vi "数据采集传输系统.vi"() -> ()   [LabVIEW 2016, in "数据传输系统.lvlib"]
uses:
  <vilib>/Utility/miscctls.llb/LVPointTypeDef.ctl
  <vilib>/Utility/config.llb/Read Key (String).vi
  <vilib>/Utility/config.llb/Read Key (Boolean).vi
  <vilib>/Utility/config.llb/Read Key (I32).vi
  <vilib>/Utility/config.llb/Write Key (String).vi
  <vilib>/Utility/config.llb/Write Key (U32).vi
  <vilib>/Utility/config.llb/Write Key (Boolean).vi
  <vilib>/Utility/config.llb/Write Key (I32).vi
  <vilib>/Utility/config.llb/NI_LVConfig.lvlib
  data/FreeMem.dll
  <vilib>/ptbypt/NI_PtbyPt.lvlib
panel:
  in  "实时数据发送时间间隔/min":i32=1
  in  "数据组合发送":bool
  in  "日志、参数发送":bool
  in  "2011发送":bool
  in  "判断数据反馈":bool
  in  "数据发送协议":enum16{"2005-212协议", "2017-212协议"}(ring)=enum."2017-212协议"
  in  "数据发送通道":enum16{"TCP", "VISA"}(ring)
  in  "baud rate":u32=9600 caption="波特率"
  in  "VISA resource name":refnum<visa-resource-name> caption="VISA资源名称"
  in  "查询质控数据起始时间":bool
  in  "返回主界面":bool
  out "零点核查索引起始时间":string
  out "跨度核查索引起始时间":string
  out "加标回收索引起始时间":string
  out "标样核查索引起始时间":string
  out "数据接收超时指示灯":bool
  in  "重发时间":T1(ring)
  in  "重发日期":T2(ring)
  in  "锁":bool
  in  "开机启动":bool
  in  "确定更改起始时间":bool
  in  "更改起始时间":bool
  in  "数据发送起始时间":timestamp format="%<%.3X\n%Y/%m/%d>T"
  in  "每周自动重发":bool=TRUE
  in  "确定":bool
  in  "返回":bool
  in  "PW":string
  in  "MN":string
  in  "PORT":string
  in  "IP":string
  in  "站点设备":string
  in  "站点名称":string
  out "设置超时时间/min":i32=1
  out "空闲时间/s":string
  out "状态信息":T3={"1st Error to Convert "=63, "步骤 "=enum."打开连接", "元素"="实时数据", "TCP服务端掉线计数"=4, "TCP掉线时间节点"="2019/05/08 15:24:17"} {"1st Error to Convert" items=["无错误", "参数错误", "内存已满", "超出区域", "文件结束", "文件已打开", "一般文件IO错误", "未找到文件", "文件权限错误", "磁盘已满", "路径副本", "打开过多文件", "未启用", "未找到资源文件", "无法添加资源", "未找到资源", "未找到图像", "图像内存错误", "画笔不存在", "配置错误类型", "配置未找到解析段", "配置解析错误", "配置内存错误", "错误外部代码格式", "错误外部代码偏移量", "外部代码不存在", "空窗口", "销毁窗口错误", "空菜单", "打印已中止", "错误打印记录", "打印驱动程序错误", "打印时窗口错误", "打印时内存错误", "打印对话框错误", "一般打印错误", "无效设备引用句柄", "设备未找到", "设备参数错误", "设备单位错误", "无法打开设备", "设备调用已中止", "一般错误", "用户已取消", "对象ID过低", "对象ID过高", "对象不在堆中", "未知的堆", "错误DefProc ID", "DefProc不在表格中", "范围外信息", "空方法", "未知信息", "不支持管理器调用", "错误地址", "连接过程中", "连接超时", "连接过程中", "不支持网络属性", "网络错误", "正在使用的地址", "系统缺少内存", "连接已中止", "连接已拒绝", "连接未建立", "连接已建立", "连接已关闭", "初始化错误（交互应用程序管理器）", "错误事件发生", "等待无约束事件发生处理程序", "事件发生队列溢出", "错误路径", "未发出信号量", "未识别类型（交互应用程序管理器）"]}
  out "系统时间":string
  out "实时小时数据上传":bool
  out "系统状态改变":bool
  out "软件版本":string
  out "掉线指示":bool
  out "核查数据上传":bool
  out "通信状态":bool
  out "配置信息":T4
  in  "参数配置":bool
  out "查询数据发送":bool
  out "读取报文显示":string
  out "发送报文显示":string
  out "心跳包":bool
  in  "参数数值":T5={"CODMn"=TRUE, "CODCr"=TRUE, "DO"=TRUE, "铜"=TRUE, "PH"=TRUE, "氨氮"=TRUE, "比电导率"=TRUE, "水温"=TRUE, "盐度(海水)"=TRUE, "浊度"=TRUE, "总氮"=TRUE, "总磷"=TRUE, "叶绿素a"=TRUE, "藻密度"=TRUE, "水位"=TRUE, "流速"=TRUE, "瞬时流量"=TRUE, "累积流量"=TRUE}
  in  "系统编码选择框":string(combo)="地表水质量监测"
  out "主队列输出":refnum<queue>
  in  "TCP掉线时间节点":string
  out "TCP服务端掉线计数":i32
  out "元素":string
  out "步骤":T6(ring)
  out "1st Error to Convert":i32(ring)=56 items=["无错误", "参数错误", "内存已满", "超出区域", "文件结束", "文件已打开", "一般文件IO错误", "未找到文件", "文件权限错误", "磁盘已满", "路径副本", "打开过多文件", "未启用", "未找到资源文件", "无法添加资源", "未找到资源", "未找到图像", "图像内存错误", "画笔不存在", "配置错误类型", "配置未找到解析段", "配置解析错误", "配置内存错误", "错误外部代码格式", "错误外部代码偏移量", "外部代码不存在", "空窗口", "销毁窗口错误", "空菜单", "打印已中止", "错误打印记录", "打印驱动程序错误", "打印时窗口错误", "打印时内存错误", "打印对话框错误", "一般打印错误", "无效设备引用句柄", "设备未找到", "设备参数错误", "设备单位错误", "无法打开设备", "设备调用已中止", "一般错误", "用户已取消", "对象ID过低", "对象ID过高", "对象不在堆中", "未知的堆", "错误DefProc ID", "DefProc不在表格中", "范围外信息", "空方法", "未知信息", "不支持管理器调用", "错误地址", "连接过程中", "连接超时", "连接过程中", "不支持网络属性", "网络错误", "正在使用的地址", "系统缺少内存", "连接已中止", "连接已拒绝", "连接未建立", "连接已建立", "连接已关闭", "初始化错误（交互应用程序管理器）", "错误事件发生", "等待无约束事件发生处理程序", "事件发生队列溢出", "错误路径", "未发出信号量", "未识别类型（交互应用程序管理器）"]
  out "QN":string
  out "时间QN":string
  out "系统编码ST":string
  out "命令编码CN":string
  out "密码PW":string
  out "设备编码MN":string
  out "拆分包及应答Flag":string
  out "数据":string
  in  "实时数据参数选择框":T7={"水样测量数据"=FALSE, "零点核查数据"=TRUE, "跨度核查数据"=TRUE, "加标回收数据"=TRUE, "平行样数据"=FALSE, "标样核查"=TRUE, "集成干预测试"=TRUE}
  out "数据输出":string
  in  "table元素":string
  out "空闲时间":dbl
  # "数 据 采 集 传 输 系 统"
  # "读取的参数区"
  # "水样测量数据"
  # "空白测试数据"
  # "跨度核查数据"
  # "加标回收数据"
  # "平行样数据"
  # "标样核查"
  # "集成干预测试"
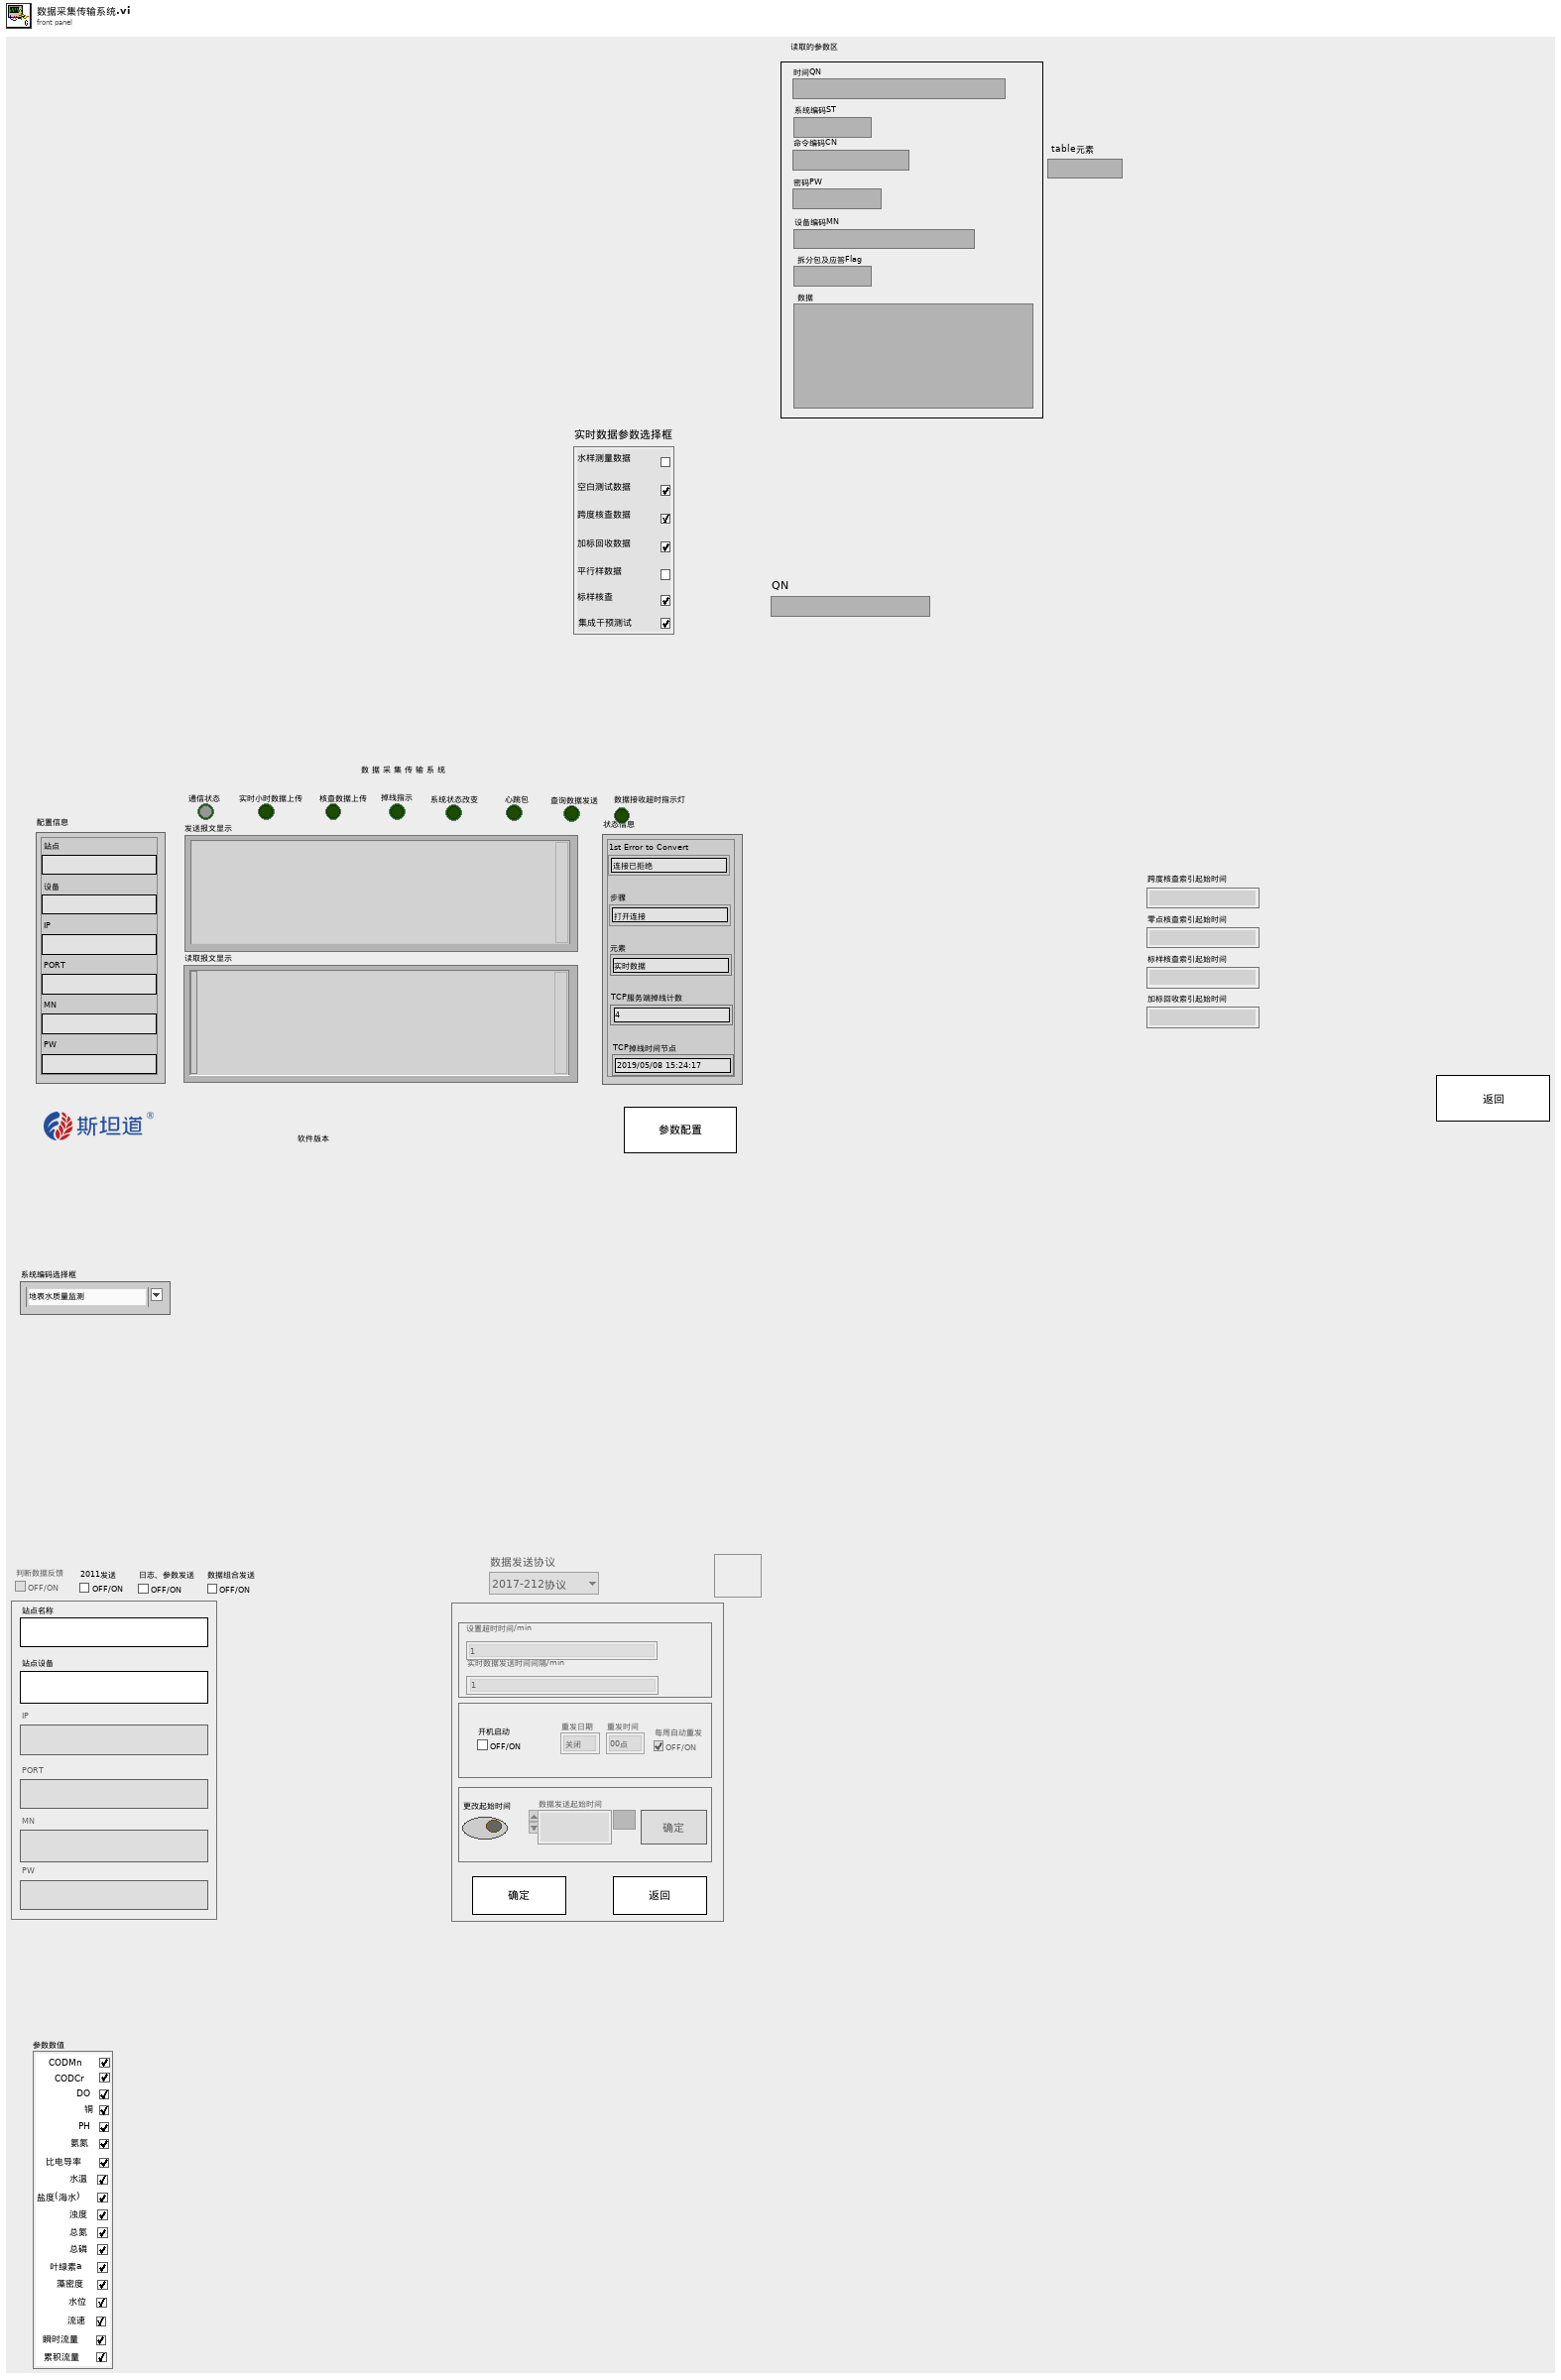
[diagram p1: front panel]
types:
  T1 = enum16{"00点", "01点", "02点", "03点", "04点", "05点", "06点", "07点", "08点", "09点", "10点", "11点", "12点", "13点", "14点", "15点", "16点", "17点", "18点", "19点", "20点", "21点", "22点", "23点"}
  T2 = enum16{"关闭", "星期日", "星期一", "星期二", "星期三", "星期四", "星期五", "星期六"}
  T3 = cluster{"1st Error to Convert ":i32, "步骤 ":enum16{"初始化", "打开连接", "表格比对", "发送数据", "读取数据", "数据处理"}, "元素":string, "TCP服务端掉线计数":i32, "TCP掉线时间节点":string}
  T4 = cluster{"站点":string, "设备":string, "IP":string, "PORT":string, "MN":string, "PW":string}
  T5 = cluster{"CODMn":bool, "CODCr":bool, "DO":bool, "铜":bool, "PH":bool, "氨氮":bool, "比电导率":bool, "水温":bool, "盐度(海水)":bool, "浊度":bool, "总氮":bool, "总磷":bool, "叶绿素a":bool, "藻密度":bool, "水位":bool, "流速":bool, "瞬时流量":bool, "累积流量":bool}
  T6 = enum16{"初始化", "打开连接", "表格比对", "发送数据", "读取数据", "数据处理"}
  T7 = cluster{"水样测量数据":bool, "零点核查数据":bool, "跨度核查数据":bool, "加标回收数据":bool, "平行样数据":bool, "标样核查":bool, "集成干预测试":bool}
  T8 = typedef "NI_LVConfig.lvlib/Config Data RefNum.ctl" = refnum<k1>
  T9 = typedef "LVDateTimeRec.ctl" = cluster{"秒数的小数部分":dbl, "秒":i32, "分":i32, "时":i32, "日":i32, "月":i32, "年":i32, "天数（周）":i32, "天数（年）":i32, "DST":i32}
  T10 = enum8{"Enabled", "Disabled", "Disabled and Grayed Out"}
  T11 = typedef "LVPointTypeDef.ctl" = cluster{"Horizontal":i16, "Vertical":i16}
  T12 = enum16{"水样测试", "小时数据", "日志信息", "报警信息", "零点核查", "标样核查", "平行样", "加标回收"}
  T13 = typedef "imagedata.ctl" = cluster{"image type":i32, "image depth":i32, "image":u8[], "mask":u8[], "colors":u32[], "Rectangle":cluster{"left":i16, "top":i16, "right":i16, "bottom":i16}}
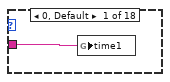
[diagram p5: hidden frame]
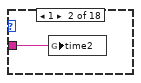
[diagram p6: hidden frame]
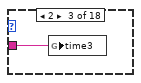
[diagram p7: hidden frame]
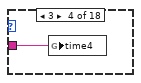
[diagram p8: hidden frame]
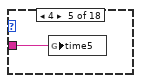
[diagram p9: hidden frame]
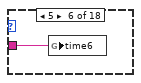
[diagram p10: hidden frame]
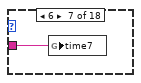
[diagram p11: hidden frame]
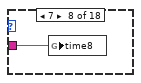
[diagram p12: hidden frame]
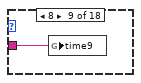
[diagram p13: hidden frame]
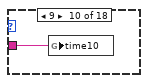
[diagram p14: hidden frame]
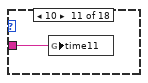
[diagram p15: hidden frame]
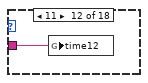
[diagram p16: hidden frame]
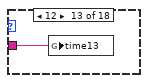
[diagram p17: hidden frame]
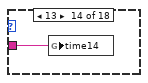
[diagram p18: hidden frame]
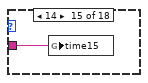
[diagram p19: hidden frame]
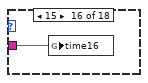
[diagram p20: hidden frame]
diagram:
  w36 = 0 ("索引")
  # "上传本地时间点的实时数据"
  # "目前时间太短，如果掉线了，数据存不了临时表格"
  n1 = Cluster To Array(cluster="参数数值") -> (array=w47:bool[])
  n2 = for {
    tunnel: w47 -> [_] mode=indexing
    tunnel: [w74] -> w46
    i -> [w74]
    w63 = "线程一数据重发功能" ("section")
    # "初始化水样搜索起始时间"
    n3 = case shown="3" w74 {
      tunnel: [w105 w107 w109 w111 w113 w115 w117 w119 w121 w123 w125 w127 w129 w131 w133 w135 w137 w139] -> w78
      frame 0, Default {
        n4 = control-ref of="CODMn"() -> (w106:refnum<vi>)
        n5 = property class="Bool (严格)"(reference=w106) -> ("Label.Text"=w105:string)  [unwired: 1 in, 2 out]
      }
      frame 1 {
        n6 = control-ref of="CODCr"() -> (w108:refnum<vi>)
        n7 = property class="Bool (严格)"(reference=w108) -> ("Label.Text"=w107:string)  [unwired: 1 in, 2 out]
      }
      frame 2 {
        n8 = control-ref of="DO"() -> (w110:refnum<vi>)
        n9 = property class="Bool (严格)"(reference=w110) -> ("Label.Text"=w109:string)  [unwired: 1 in, 2 out]
      }
      frame 3 {
        n10 = control-ref of="铜"() -> (w112:refnum<vi>)
        n11 = property class="Bool (严格)"(reference=w112) -> ("Label.Text"=w111:string)  [unwired: 1 in, 2 out]
      }
      frame 4 {
        n12 = control-ref of="PH"() -> (w114:refnum<vi>)
        n13 = property class="Bool (严格)"(reference=w114) -> ("Label.Text"=w113:string)  [unwired: 1 in, 2 out]
      }
      frame 5 {
        n14 = control-ref of="氨氮"() -> (w116:refnum<vi>)
        n15 = property class="Bool (严格)"(reference=w116) -> ("Label.Text"=w115:string)  [unwired: 1 in, 2 out]
      }
      frame 6 {
        n16 = control-ref of="比电导率"() -> (w118:refnum<vi>)
        n17 = property class="Bool (严格)"(reference=w118) -> ("Label.Text"=w117:string)  [unwired: 1 in, 2 out]
      }
      frame 7 {
        n18 = control-ref of="水温"() -> (w120:refnum<vi>)
        n19 = property class="Bool (严格)"(reference=w120) -> ("Label.Text"=w119:string)  [unwired: 1 in, 2 out]
      }
      frame 8 {
        n20 = control-ref of="盐度(海水)"() -> (w122:refnum<vi>)
        n21 = property class="Bool (严格)"(reference=w122) -> ("Label.Text"=w121:string)  [unwired: 1 in, 2 out]
      }
      frame 9 {
        n22 = control-ref of="浊度"() -> (w124:refnum<vi>)
        n23 = property class="Bool (严格)"(reference=w124) -> ("Label.Text"=w123:string)  [unwired: 1 in, 2 out]
      }
      frame 10 {
        n24 = control-ref of="总氮"() -> (w126:refnum<vi>)
        n25 = property class="Bool (严格)"(reference=w126) -> ("Label.Text"=w125:string)  [unwired: 1 in, 2 out]
      }
      frame 11 {
        n26 = control-ref of="总磷"() -> (w128:refnum<vi>)
        n27 = property class="Bool (严格)"(reference=w128) -> ("Label.Text"=w127:string)  [unwired: 1 in, 2 out]
      }
      frame 12 {
        n28 = control-ref of="叶绿素a"() -> (w130:refnum<vi>)
        n29 = property class="Bool (严格)"(reference=w130) -> ("Label.Text"=w129:string)  [unwired: 1 in, 2 out]
      }
      frame 13 {
        n30 = control-ref of="藻密度"() -> (w132:refnum<vi>)
        n31 = property class="Bool (严格)"(reference=w132) -> ("Label.Text"=w131:string)  [unwired: 1 in, 2 out]
      }
      frame 14 {
        n32 = control-ref of="水位"() -> (w134:refnum<vi>)
        n33 = property class="Bool (严格)"(reference=w134) -> ("Label.Text"=w133:string)  [unwired: 1 in, 2 out]
      }
      frame 15 {
        n34 = control-ref of="流速"() -> (w136:refnum<vi>)
        n35 = property class="Bool (严格)"(reference=w136) -> ("Label.Text"=w135:string)  [unwired: 1 in, 2 out]
      }
      frame 16 {
        n36 = control-ref of="瞬时流量"() -> (w138:refnum<vi>)
        n37 = property class="Bool (严格)"(reference=w138) -> ("Label.Text"=w137:string)  [unwired: 1 in, 2 out]
      }
      frame 17 {
        n38 = control-ref of="累积流量"() -> (w140:refnum<vi>)
        n39 = property class="Bool (严格)"(reference=w140) -> ("Label.Text"=w139:string)  [unwired: 1 in, 2 out]
      }
    }
    n40 = call <vilib>:"Application Directory.vi"() -> ("Application Directory"=w84:path)
    n41 = Build Path(base path=w84, name or relative path="data\\Set.ini" ("名称或相对路径")) -> (appended path=w82:path)
    n42 = call <vilib>:"Open Config Data.vi"("configuration file path"=w82) -> ("error out"=w80:errorcluster, "refnum"=w81:T8)  [unwired: 8 in, 1 out]
    n43 = call-poly <vilib>:"Read Key.vi"("section"="线程一数据搜索起始时间", "error in (no error)"=w80, "key"=w78, "refnum"=w81) -> ("error out"=w72:errorcluster, "value"=w75:string, "refnum out"=w73:T8)  [unwired: 4 in, 1 out]
    n44 = Empty String/Path?(string/path=w75) -> (empty?=w77:bool)
    n45 = case shown="真" w77 {
      tunnel: [w85 "1904/01/01 00:00:00"] -> w76
      tunnel: w75 -> [w85 _]
      frame False {
      }
      frame True {
      }
    }
    n46 = call-poly <vilib>:"Read Key.vi"("section"=w63, "error in (no error)"=w72, "key"="重发功能", "refnum"=w73) -> ("error out"=w66:errorcluster, "value"=w70:bool, "refnum out"=w67:T8)  [unwired: 4 in, 1 out]
    n47 = local write "每周自动重发"(w70) -> ()
    n48 = call-poly <vilib>:"Read Key.vi"("section"=w63, "error in (no error)"=w66, "key"="重发日期", "refnum"=w67) -> ("error out"=w64:errorcluster, "value"=w60:i32, "refnum out"=w65:T8)  [unwired: 4 in, 1 out]
    n49 = local write "重发日期"(w60) -> ()
    n50 = case shown="3" w74 {
      tunnel: w76 -> [w87 w88 w89 w90 w91 w92 w93 w94 w95 w96 w97 w98 w99 w100 w101 w102 w103 w104]
      frame 0, Default {
        n51 = global write "全局 水样时间.vi" "time1"(w87) -> ()
      }
      frame 1 {
        n52 = global write "全局 水样时间.vi" "time2"(w88) -> ()
      }
      frame 2 {
        n53 = global write "全局 水样时间.vi" "time3"(w89) -> ()
      }
      frame 3 {
        n54 = global write "全局 水样时间.vi" "time4"(w90) -> ()
      }
      frame 4 {
        n55 = global write "全局 水样时间.vi" "time5"(w91) -> ()
      }
      frame 5 {
        n56 = global write "全局 水样时间.vi" "time6"(w92) -> ()
      }
      frame 6 {
        n57 = global write "全局 水样时间.vi" "time7"(w93) -> ()
      }
      frame 7 {
        n58 = global write "全局 水样时间.vi" "time8"(w94) -> ()
      }
      frame 8 {
        n59 = global write "全局 水样时间.vi" "time9"(w95) -> ()
      }
      frame 9 {
        n60 = global write "全局 水样时间.vi" "time10"(w96) -> ()
      }
      frame 10 {
        n61 = global write "全局 水样时间.vi" "time11"(w97) -> ()
      }
      frame 11 {
        n62 = global write "全局 水样时间.vi" "time12"(w98) -> ()
      }
      frame 12 {
        n63 = global write "全局 水样时间.vi" "time13"(w99) -> ()
      }
      frame 13 {
        n64 = global write "全局 水样时间.vi" "time14"(w100) -> ()
      }
      frame 14 {
        n65 = global write "全局 水样时间.vi" "time15"(w101) -> ()
      }
      frame 15 {
        n66 = global write "全局 水样时间.vi" "time16"(w102) -> ()
      }
      frame 16 {
        n67 = global write "全局 水样时间.vi" "time17"(w103) -> ()
      }
      frame 17 {
        n68 = global write "全局 水样时间.vi" "time18"(w104) -> ()
      }
    }
    n69 = call-poly <vilib>:"Read Key.vi"("section"=w63, "error in (no error)"=w64, "key"="重发时间", "refnum"=w65) -> ("error out"=w61:errorcluster, "value"=w59:i32, "refnum out"=w62:T8)  [unwired: 4 in, 1 out]
    n70 = local write "重发时间"(w59) -> ()
    n71 = call <vilib>:"Close Config Data.vi"("error in (no error)"=w61, "refnum"=w62) -> ()  [unwired: 8 in, 2 out]
  }
  n72 = vi-ref "数据传输系统.lvlib:核查数据和日志信息入发送队列 (子VI).vi"() -> (w19:refnum<vi>)
  n73 = vi-ref "数据传输系统.lvlib:主动上传工控机周期和模式 (子VI).vi"() -> (w28:refnum<vi>)
  n74 = vi-ref "数据传输系统.lvlib:核查数据和日志信息出发送队列 (子VI).vi"() -> (w10:refnum<vi>)
  n75 = local read "实时小时数据上传"() -> (w15:bool)
  n76 = property class="VI"(reference=w28) -> ("Name"=w29:string)  [unwired: 1 in, 2 out]
  n77 = property class="VI"(reference=w10) -> ("Name"=w9:string)  [unwired: 1 in, 2 out]
  n78 = local read "查询数据发送"() -> (w2:bool)
  n79 = local read "核查数据上传"() -> (w18:bool)
  n80 = local read "查询数据发送"() -> (w17:bool)
  n81 = local read "日志、参数发送"() -> (w13:bool)
  n82 = property class="VI"(reference=w19) -> ("Name"=w26:string)  [unwired: 1 in, 2 out]
  n83 = local read "步骤"() -> (w16:T6)
  n84 = local read "数据发送协议"() -> (w14:enum16{"2005-212协议", "2017-212协议"})
  n85 = Open VI Reference(type specifier VI Refnum (for type only)=refnum<vi> refnum, vi path=w29, options=128 ("选项")) -> (vi reference=w31:refnum<vi>, error out=w33:errorcluster)  [unwired: 3 in]
  n86 = Open VI Reference(type specifier VI Refnum (for type only)=refnum<vi> refnum, vi path=w9, options=128 ("选项")) -> (vi reference=w7:refnum<vi>, error out=w5:errorcluster)  [unwired: 3 in]
  n87 = Open VI Reference(type specifier VI Refnum (for type only)=refnum<vi> refnum, vi path=w26, options=128 ("选项")) -> (vi reference=w24:refnum<vi>, error out=w22:errorcluster)  [unwired: 3 in]
  n88 = call-by-ref "?"(reference=w31, error in=w33) -> (reference out=w35:refnum<vi>, error out=w34:errorcluster, "系统状态改变"=→"系统状态改变":bool)  [unwired: 11 in]
  n89 = call-by-ref "?"(reference=w7, error in=w5, "查询数据发送"=w2) -> (reference out=w3:refnum<vi>, error out=w4:errorcluster, "核查数据上传"=→"核查数据上传":bool)  [unwired: 10 in]
  n90 = call-by-ref "?"(reference=w24, error in=w22, "实时数据参数选择框"="实时数据参数选择框", "实时数据发送时间间隔/min"="实时数据发送时间间隔/min", "日志、参数发送输入"=w13, "数据发送协议输入"=w14, "实时小时数据上传输入"=w15, "步骤输入"=w16, "查询数据发送输入"=w17, "核查数据上传输入"=w18) -> (reference out=w20:refnum<vi>, error out=w21:errorcluster)  [unwired: 4 in]
  n91 = Close Reference(reference=w35, error in (no error)=w34) -> ()  [unwired: 1 out]
  n92 = Close Reference(reference=w3, error in (no error)=w4) -> ()  [unwired: 1 out]
  n93 = Close Reference(reference=w20, error in (no error)=w21) -> ()  [unwired: 1 out]
  n94 = while "While循环" {
    tunnel: [w155] -> _
    tunnel: w46 -> [w149]
    stop <- FALSE stop-if-true
    w143 = FALSE ("小时数据上传")
    # "2017，2005版协议实时、小时数据出数据就单参数上传"
    n95 = property on="TCP服务端掉线计数" class="DigNum (严格)"() -> ("Value"=w152:i32)  [unwired: 2 in, 2 out]
    n96 = local read "查询数据发送"() -> (w145:bool)
    n97 = local read "核查数据上传"() -> (w144:bool)
    n98 = local read "步骤"() -> (w154:T6)
    n99 = local write "实时小时数据上传"(w143) -> ()
    n100 = global write "全局 数据发送重叠.vi" "主动上报数据中"(w143) -> ()
    n101 = Greater Or Equal?(x=w149, y=17) -> (x >= y?=w148:bool)
    n102 = Equal To 0?(x=w152) -> (x = 0?=w150:bool)
    n103 = Not(x=w145) -> (.not. x?=w142:bool)
    n104 = Not(x=w144) -> (.not. x?=w141:bool)
    n105 = Equal?(x=w154, y=T6."读取数据" ("步骤")) -> (x = y?=w151:bool)
    n106 = Wait (ms)(milliseconds to wait=u32 75430 ("等待时间（毫秒）")) -> ()  [unwired: 1 out]
    n107 = Compound Arithmetic op=AND ("复合运算")(w151, w150, w148, w142, w141) -> (w146:bool)
    n108 = case shown="真" w146 {
      tunnel: [_ w160] -> w155
      frame False {
        w158 = FALSE ("小时数据上传")
        n109 = local write "实时小时数据上传"(w158) -> ()
        n110 = global write "全局 数据发送重叠.vi" "主动上报数据中"(w158) -> ()
      }
      frame True {
        n111 = global read "断电保存全局.vi" "数据组合发送"() -> (w159:bool)
        n112 = case shown="假" w159 {
          tunnel: [w161 _] -> w160
          frame False {
            # "数据非整点触发，而是实时触发，分条发送"
            n113 = flat-sequence {
              tunnel: [w165] -> w162
              tunnel: [w446] -> w161
              tunnel: w162 -> [w446]
              frame #0 {
                w163 = TRUE ("小时数据上传")
                n114 = global write "全局 数据发送重叠.vi" "主动上报数据中"(w163) -> ()
                n115 = local read "数据发送协议"() -> (w164:enum16{"2005-212协议", "2017-212协议"})
                n116 = case shown="\"2005-212协议\"" w164 {
                  tunnel: [_ w267] -> w165
                  frame "2005-212协议" {
                    n117 = local read "参数数值"() -> (w169:T5)
                    n118 = Cluster To Array(cluster=w169) -> (array=w168:bool[])
                    n119 = for {
                      tunnel: w168 -> [_] mode=indexing
                      tunnel: [w212] -> w167
                      i -> [w210]
                      (unwired) " where 时间 between #"
                      w208 = "database1.mdb" ("database")
                      (unwired) "'and 数据类型 ='N' and 时间 between "
                      n120 = case shown="12" w210 {
                        tunnel: [w231 w233 w235 w237 w239 w241 w243 w245 w247 w249 w251 w253 w255 w257 w259 w261 w263 w265] -> w209
                        frame 0, Default {
                          n121 = control-ref of="CODMn"() -> (w232:refnum<vi>)
                          n122 = property class="Bool (严格)"(reference=w232) -> ("Label.Text"=w231:string)  [unwired: 1 in, 2 out]
                        }
                        frame 1 {
                          n123 = control-ref of="CODCr"() -> (w234:refnum<vi>)
                          n124 = property class="Bool (严格)"(reference=w234) -> ("Label.Text"=w233:string)  [unwired: 1 in, 2 out]
                        }
                        frame 2 {
                          n125 = control-ref of="DO"() -> (w236:refnum<vi>)
                          n126 = property class="Bool (严格)"(reference=w236) -> ("Label.Text"=w235:string)  [unwired: 1 in, 2 out]
                        }
                        frame 3 {
                          n127 = control-ref of="铜"() -> (w238:refnum<vi>)
                          n128 = property class="Bool (严格)"(reference=w238) -> ("Label.Text"=w237:string)  [unwired: 1 in, 2 out]
                        }
                        frame 4 {
                          n129 = control-ref of="PH"() -> (w240:refnum<vi>)
                          n130 = property class="Bool (严格)"(reference=w240) -> ("Label.Text"=w239:string)  [unwired: 1 in, 2 out]
                        }
                        frame 5 {
                          n131 = control-ref of="氨氮"() -> (w242:refnum<vi>)
                          n132 = property class="Bool (严格)"(reference=w242) -> ("Label.Text"=w241:string)  [unwired: 1 in, 2 out]
                        }
                        frame 6 {
                          n133 = control-ref of="比电导率"() -> (w244:refnum<vi>)
                          n134 = property class="Bool (严格)"(reference=w244) -> ("Label.Text"=w243:string)  [unwired: 1 in, 2 out]
                        }
                        frame 7 {
                          n135 = control-ref of="水温"() -> (w246:refnum<vi>)
                          n136 = property class="Bool (严格)"(reference=w246) -> ("Label.Text"=w245:string)  [unwired: 1 in, 2 out]
                        }
                        frame 8 {
                          n137 = control-ref of="盐度(海水)"() -> (w248:refnum<vi>)
                          n138 = property class="Bool (严格)"(reference=w248) -> ("Label.Text"=w247:string)  [unwired: 1 in, 2 out]
                        }
                        frame 9 {
                          n139 = control-ref of="浊度"() -> (w250:refnum<vi>)
                          n140 = property class="Bool (严格)"(reference=w250) -> ("Label.Text"=w249:string)  [unwired: 1 in, 2 out]
                        }
                        frame 10 {
                          n141 = control-ref of="总氮"() -> (w252:refnum<vi>)
                          n142 = property class="Bool (严格)"(reference=w252) -> ("Label.Text"=w251:string)  [unwired: 1 in, 2 out]
                        }
                        frame 11 {
                          n143 = control-ref of="总磷"() -> (w254:refnum<vi>)
                          n144 = property class="Bool (严格)"(reference=w254) -> ("Label.Text"=w253:string)  [unwired: 1 in, 2 out]
                        }
                        frame 12 {
                          n145 = control-ref of="叶绿素a"() -> (w256:refnum<vi>)
                          n146 = property class="Bool (严格)"(reference=w256) -> ("Label.Text"=w255:string)  [unwired: 1 in, 2 out]
                        }
                        frame 13 {
                          n147 = control-ref of="藻密度"() -> (w258:refnum<vi>)
                          n148 = property class="Bool (严格)"(reference=w258) -> ("Label.Text"=w257:string)  [unwired: 1 in, 2 out]
                        }
                        frame 14 {
                          n149 = control-ref of="水位"() -> (w260:refnum<vi>)
                          n150 = property class="Bool (严格)"(reference=w260) -> ("Label.Text"=w259:string)  [unwired: 1 in, 2 out]
                        }
                        frame 15 {
                          n151 = control-ref of="流速"() -> (w262:refnum<vi>)
                          n152 = property class="Bool (严格)"(reference=w262) -> ("Label.Text"=w261:string)  [unwired: 1 in, 2 out]
                        }
                        frame 16 {
                          n153 = control-ref of="瞬时流量"() -> (w264:refnum<vi>)
                          n154 = property class="Bool (严格)"(reference=w264) -> ("Label.Text"=w263:string)  [unwired: 1 in, 2 out]
                        }
                        frame 17 {
                          n155 = control-ref of="累积流量"() -> (w266:refnum<vi>)
                          n156 = property class="Bool (严格)"(reference=w266) -> ("Label.Text"=w265:string)  [unwired: 1 in, 2 out]
                        }
                      }
                      n157 = global read "断电保存全局.vi" "数据发送协议"() -> (w206:enum16{"2005-212协议", "2017-212协议"})
                      n158 = call "主动发送数据生成Condition(子VI).vi"("数据发送协议"=w206, "database"=w208, "Label.Text"=w209, "数值"=w210) -> ("CONDITION"=w207:string)  [unwired: 7 in]
                      n159 = call "SQL查询.vi"("condition"=w207, "table输入"=w209, "database"=w208) -> ("error out"=w212:errorcluster, "data"=w211:string[][])  [unwired: 7 in]
                      n160 = case shown="3" w210 {
                        tunnel: w211 -> [w213 w214 w215 w216 w217 w218 w219 w220 w221 w222 w223 w224 w225 w226 w227 w228 w229 w230]
                        frame 0, Default {
                          n161 = global write "全局 所有参数.vi" "CODMn"(w213) -> ()
                        }
                        frame 1 {
                          n162 = global write "全局 所有参数.vi" "CODCr"(w214) -> ()
                        }
                        frame 2 {
                          n163 = global write "全局 所有参数.vi" "DO"(w215) -> ()
                        }
                        frame 3 {
                          n164 = global write "全局 所有参数.vi" "铜"(w216) -> ()
                        }
                        frame 4 {
                          n165 = global write "全局 所有参数.vi" "PH"(w217) -> ()
                        }
                        frame 5 {
                          n166 = global write "全局 所有参数.vi" "氨氮"(w218) -> ()
                        }
                        frame 6 {
                          n167 = global write "全局 所有参数.vi" "电导率"(w219) -> ()
                        }
                        frame 7 {
                          n168 = global write "全局 所有参数.vi" "水温"(w220) -> ()
                        }
                        frame 8 {
                          n169 = global write "全局 所有参数.vi" "盐度"(w221) -> ()
                        }
                        frame 9 {
                          n170 = global write "全局 所有参数.vi" "浊度"(w222) -> ()
                        }
                        frame 10 {
                          n171 = global write "全局 所有参数.vi" "总氮"(w223) -> ()
                        }
                        frame 11 {
                          n172 = global write "全局 所有参数.vi" "总磷"(w224) -> ()
                        }
                        frame 12 {
                          n173 = global write "全局 所有参数.vi" "叶绿素"(w225) -> ()
                        }
                        frame 13 {
                          n174 = global write "全局 所有参数.vi" "藻密度"(w226) -> ()
                        }
                        frame 14 {
                          n175 = global write "全局 所有参数.vi" "水位"(w227) -> ()
                        }
                        frame 15 {
                          n176 = global write "全局 所有参数.vi" "流速"(w228) -> ()
                        }
                        frame 16 {
                          n177 = global write "全局 所有参数.vi" "瞬时流量"(w229) -> ()
                        }
                        frame 17 {
                          n178 = global write "全局 所有参数.vi" "累积流量"(w230) -> ()
                        }
                      }
                    }
                    n179 = flat-sequence {
                      tunnel: w167 -> [w170]
                      tunnel: [w170] -> w166
                      tunnel: w166 -> [w176]
                      tunnel: [w175] -> _
                      frame #0 {
                        n180 = global write "全局 小时数据发送次数.vi" "小时数据发送次数"(0 ("小时数据发送次数")) -> ()
                        n181 = call "数据处理直接插入整合 (子VI).vi"() -> ()  [unwired: 12 in]
                        n182 = global write "全局1.vi" "枚举"(enum16{"返回请求应答", "上传数据", "返回执行结果"}."上传数据" ("枚举")) -> ()
                        n183 = global write "全局 实时数据参数.vi" "实时数据参数"("水样测试" ("实时数据参数")) -> ()
                        n184 = global write "全局 水样时间.vi" "选择发送的参数"("氨氮" ("选择发送的参数")) -> ()
                      }
                      frame #1 {
                        # "实时数据的大小"
                        n185 = flat-sequence {
                          tunnel: [w180] -> w179
                          tunnel: [w185] -> w177
                          tunnel: w176 -> [w184]
                          tunnel: w179 -> [_]
                          tunnel: [w195] -> w178
                          tunnel: w177 -> [w195]
                          tunnel: w178 -> [w203]
                          tunnel: [w201] -> w175
                          frame #0 {
                            n186 = Get Date/Time In Seconds() -> (seconds since 1Jan1904=w190:timestamp)
                            n187 = Format Date/Time String(time format string (%c)="%Y%m%d%H%M%S%3u" ("时间格式字符串(%c)"), seconds (now)=w190) -> (date/time string=w191:string)  [unwired: 1 in]
                            n188 = Search and Replace String(input string=w191, search string="." ("搜索字符串")) -> (result string=w193:string)  [unwired: 6 in, 3 out]
                            n189 = global read "全局1.vi" "MN"() -> (w182:string)
                            n190 = global read "全局1.vi" "PW"() -> (w181:string)
                            n191 = global read "断电保存全局.vi" "数据发送通道"() -> (w183:enum16{"TCP", "VISA"})
                            n192 = call "数据编码.vi"("table输入"="小时数据" ("新元素/子数组"), "QN"=w193, "MN"=w182, "PW"=w181) -> ("通讯包字符串"=w180:string)  [unwired: 10 in, 1 out]
                            n193 = Build Array(w180) -> (w187:string[])
                            n194 = global write "全局1.vi" "发送报文显示"(w180) -> ()
                            n195 = call "VISATCP组合选择发送.vi"("数据发送通道"=w183, "命令"="write", "写入缓冲区"=w180) -> ()  [unwired: 9 in, 4 out]
                            n196 = call "发送数据记录到文档(子VI).vi"("错误输入"=w184, "数组"=w187) -> ("错误输出"=w185:errorcluster)  [unwired: 8 in]
                          }
                          frame #1 {
                            n197 = global write "全局 小时数据发送次数.vi" "小时数据发送次数"(0 ("小时数据发送次数")) -> ()
                            n198 = Wait (ms)(milliseconds to wait=u32 500 ("等待时间（毫秒）")) -> ()  [unwired: 1 out]
                          }
                          frame #2 {
                            n199 = global read "全局1.vi" "MN"() -> (w199:string)
                            n200 = global read "全局1.vi" "PW"() -> (w198:string)
                            n201 = global read "断电保存全局.vi" "数据发送通道"() -> (w200:enum16{"TCP", "VISA"})
                            n202 = call "数据编码.vi"("table输入"="实时数据" ("新元素/子数组"), "错误常量 2"=w203, "MN"=w199, "PW"=w198) -> ("通讯包字符串"=w197:string)  [unwired: 10 in, 1 out]
                            n203 = Build Array(w197) -> (w205:string[])
                            n204 = global write "全局1.vi" "发送报文显示"(w197) -> ()
                            n205 = call "发送数据记录到文档(子VI).vi"("数组"=w205) -> ()  [unwired: 9 in, 1 out]
                            n206 = call "VISATCP组合选择发送.vi"("数据发送通道"=w200, "命令"="write", "写入缓冲区"=w197) -> ("错误输出"=w201:errorcluster)  [unwired: 9 in, 3 out]
                          }
                        }
                      }
                    }
                  }
                  frame "2017-212协议", Default {
                    n207 = local read "参数数值"() -> (w269:T5)
                    n208 = Cluster To Array(cluster=w269) -> (array=w268:bool[])
                    n209 = for {
                      tunnel: w268 -> [_] mode=indexing
                      tunnel: [w274] -> w267 mode=indexing
                      tunnel: [w274] -> _
                      i -> [w273]
                      (unwired) " where 时间 between #"
                      w272 = "database1.mdb" ("database")
                      (unwired) "'and 数据类型 ='N' and 时间 between "
                      w288 = 0 ("索引 (行)")
                      n210 = case shown="3" w273 {
                        tunnel: [w409 w411 w413 w415 w417 w419 w421 w423 w425 w427 w429 w431 w433 w435 w437 w439 w441 w443] -> w271
                        frame 0, Default {
                          n211 = control-ref of="CODMn"() -> (w410:refnum<vi>)
                          n212 = property class="Bool (严格)"(reference=w410) -> ("Label.Text"=w409:string)  [unwired: 1 in, 2 out]
                        }
                        frame 1 {
                          n213 = control-ref of="CODCr"() -> (w412:refnum<vi>)
                          n214 = property class="Bool (严格)"(reference=w412) -> ("Label.Text"=w411:string)  [unwired: 1 in, 2 out]
                        }
                        frame 2 {
                          n215 = control-ref of="DO"() -> (w414:refnum<vi>)
                          n216 = property class="Bool (严格)"(reference=w414) -> ("Label.Text"=w413:string)  [unwired: 1 in, 2 out]
                        }
                        frame 3 {
                          n217 = control-ref of="铜"() -> (w416:refnum<vi>)
                          n218 = property class="Bool (严格)"(reference=w416) -> ("Label.Text"=w415:string)  [unwired: 1 in, 2 out]
                        }
                        frame 4 {
                          n219 = control-ref of="PH"() -> (w418:refnum<vi>)
                          n220 = property class="Bool (严格)"(reference=w418) -> ("Label.Text"=w417:string)  [unwired: 1 in, 2 out]
                        }
                        frame 5 {
                          n221 = control-ref of="氨氮"() -> (w420:refnum<vi>)
                          n222 = property class="Bool (严格)"(reference=w420) -> ("Label.Text"=w419:string)  [unwired: 1 in, 2 out]
                        }
                        frame 6 {
                          n223 = control-ref of="比电导率"() -> (w422:refnum<vi>)
                          n224 = property class="Bool (严格)"(reference=w422) -> ("Label.Text"=w421:string)  [unwired: 1 in, 2 out]
                        }
                        frame 7 {
                          n225 = control-ref of="水温"() -> (w424:refnum<vi>)
                          n226 = property class="Bool (严格)"(reference=w424) -> ("Label.Text"=w423:string)  [unwired: 1 in, 2 out]
                        }
                        frame 8 {
                          n227 = control-ref of="盐度(海水)"() -> (w426:refnum<vi>)
                          n228 = property class="Bool (严格)"(reference=w426) -> ("Label.Text"=w425:string)  [unwired: 1 in, 2 out]
                        }
                        frame 9 {
                          n229 = control-ref of="浊度"() -> (w428:refnum<vi>)
                          n230 = property class="Bool (严格)"(reference=w428) -> ("Label.Text"=w427:string)  [unwired: 1 in, 2 out]
                        }
                        frame 10 {
                          n231 = control-ref of="总氮"() -> (w430:refnum<vi>)
                          n232 = property class="Bool (严格)"(reference=w430) -> ("Label.Text"=w429:string)  [unwired: 1 in, 2 out]
                        }
                        frame 11 {
                          n233 = control-ref of="总磷"() -> (w432:refnum<vi>)
                          n234 = property class="Bool (严格)"(reference=w432) -> ("Label.Text"=w431:string)  [unwired: 1 in, 2 out]
                        }
                        frame 12 {
                          n235 = control-ref of="叶绿素a"() -> (w434:refnum<vi>)
                          n236 = property class="Bool (严格)"(reference=w434) -> ("Label.Text"=w433:string)  [unwired: 1 in, 2 out]
                        }
                        frame 13 {
                          n237 = control-ref of="藻密度"() -> (w436:refnum<vi>)
                          n238 = property class="Bool (严格)"(reference=w436) -> ("Label.Text"=w435:string)  [unwired: 1 in, 2 out]
                        }
                        frame 14 {
                          n239 = control-ref of="水位"() -> (w438:refnum<vi>)
                          n240 = property class="Bool (严格)"(reference=w438) -> ("Label.Text"=w437:string)  [unwired: 1 in, 2 out]
                        }
                        frame 15 {
                          n241 = control-ref of="流速"() -> (w440:refnum<vi>)
                          n242 = property class="Bool (严格)"(reference=w440) -> ("Label.Text"=w439:string)  [unwired: 1 in, 2 out]
                        }
                        frame 16 {
                          n243 = control-ref of="瞬时流量"() -> (w442:refnum<vi>)
                          n244 = property class="Bool (严格)"(reference=w442) -> ("Label.Text"=w441:string)  [unwired: 1 in, 2 out]
                        }
                        frame 17 {
                          n245 = control-ref of="累积流量"() -> (w444:refnum<vi>)
                          n246 = property class="Bool (严格)"(reference=w444) -> ("Label.Text"=w443:string)  [unwired: 1 in, 2 out]
                        }
                      }
                      n247 = global read "断电保存全局.vi" "数据发送协议"() -> (w270:enum16{"2005-212协议", "2017-212协议"})
                      n248 = call "主动发送数据生成Condition(子VI).vi"("数据发送协议"=w270, "database"=w272, "Label.Text"=w271, "数值"=w273) -> ("CONDITION"=w290:string)  [unwired: 7 in]
                      n249 = call "SQL查询.vi"("condition"=w290, "table输入"=w271, "database"=w272) -> ("error out"=w274:errorcluster, "data"=w286:string[][])  [unwired: 7 in]
                      n250 = Empty Array?(array=w286) -> (empty?=w289:bool)
                      n251 = call "短日期时间转长日期格式.vi"("data"=w286) -> ("输出数组"=w287:string[][])  [unwired: 10 in]
                      n252 = Not(x=w289) -> (.not. x?=w283:bool)
                      n253 = Index Array(array=w287, index (row)=w288, index (col)=w288) -> (element=w280:string)
                      n254 = global write "全局 水样时间.vi" "选择发送的参数"(w271) -> ()
                      n255 = flat-sequence {
                        tunnel: [w298] -> w285
                        tunnel: [w297] -> w284
                        tunnel: w283 -> [w298]
                        tunnel: w286 -> [w297]
                        tunnel: w273 -> [w292]
                        tunnel: w271 -> [w294]
                        tunnel: [w294] -> w281
                        tunnel: w280 -> [w293]
                        tunnel: [w293] -> w278
                        tunnel: [w292] -> w275
                        tunnel: w285 -> [w318]
                        tunnel: w284 -> [w321]
                        tunnel: [w320] -> w282
                        tunnel: w281 -> [w320]
                        tunnel: [w319] -> w279
                        tunnel: w278 -> [w319]
                        tunnel: [w318] -> w277
                        tunnel: [w317] -> w276
                        tunnel: w275 -> [w317]
                        tunnel: w282 -> [w377]
                        tunnel: w279 -> [w376]
                        tunnel: w277 -> [w374]
                        tunnel: w276 -> [w375]
                        frame #0 {
                          n256 = case shown="3" w292 {
                            tunnel: w297 -> [w299 w300 w301 w302 w303 w304 w305 w306 w307 w308 w309 w310 w311 w312 w313 w314 w315 w316]
                            frame 0, Default {
                              n257 = global write "全局 所有参数.vi" "CODMn"(w299) -> ()
                            }
                            frame 1 {
                              n258 = global write "全局 所有参数.vi" "CODCr"(w300) -> ()
                            }
                            frame 2 {
                              n259 = global write "全局 所有参数.vi" "DO"(w301) -> ()
                            }
                            frame 3 {
                              n260 = global write "全局 所有参数.vi" "铜"(w302) -> ()
                            }
                            frame 4 {
                              n261 = global write "全局 所有参数.vi" "PH"(w303) -> ()
                            }
                            frame 5 {
                              n262 = global write "全局 所有参数.vi" "氨氮"(w304) -> ()
                            }
                            frame 6 {
                              n263 = global write "全局 所有参数.vi" "电导率"(w305) -> ()
                            }
                            frame 7 {
                              n264 = global write "全局 所有参数.vi" "水温"(w306) -> ()
                            }
                            frame 8 {
                              n265 = global write "全局 所有参数.vi" "盐度"(w307) -> ()
                            }
                            frame 9 {
                              n266 = global write "全局 所有参数.vi" "浊度"(w308) -> ()
                            }
                            frame 10 {
                              n267 = global write "全局 所有参数.vi" "总氮"(w309) -> ()
                            }
                            frame 11 {
                              n268 = global write "全局 所有参数.vi" "总磷"(w310) -> ()
                            }
                            frame 12 {
                              n269 = global write "全局 所有参数.vi" "叶绿素"(w311) -> ()
                            }
                            frame 13 {
                              n270 = global write "全局 所有参数.vi" "藻密度"(w312) -> ()
                            }
                            frame 14 {
                              n271 = global write "全局 所有参数.vi" "水位"(w313) -> ()
                            }
                            frame 15 {
                              n272 = global write "全局 所有参数.vi" "流速"(w314) -> ()
                            }
                            frame 16 {
                              n273 = global write "全局 所有参数.vi" "瞬时流量"(w315) -> ()
                            }
                            frame 17 {
                              n274 = global write "全局 所有参数.vi" "累积流量"(w316) -> ()
                            }
                          }
                          n275 = global write "全局 小时数据发送次数.vi" "小时数据发送次数"(0 ("小时数据发送次数")) -> ()
                          n276 = global write "全局 数据发送重叠.vi" "数据接收超时指示灯"(FALSE ("数据接收超时指示灯")) -> ()
                          n277 = global write "全局1.vi" "枚举"(enum16{"返回请求应答", "上传数据", "返回执行结果"}."上传数据" ("枚举")) -> ()
                        }
                        frame #1 {
                          n278 = case shown="真" w318 {
                            tunnel: w321 -> [_ w324]
                            tunnel: w317 -> [_ w323]
                            tunnel: w317 -> [_ w322]
                            frame False {
                            }
                            frame True {
                              n279 = for {
                                tunnel: w324 -> [_] mode=indexing
                                tunnel: w323 -> [w342]
                                tunnel: w322 -> [w341]
                                # "实时数据的大小"
                                n280 = Wait (ms)(milliseconds to wait=u32 500 ("等待时间（毫秒）")) -> ()  [unwired: 1 out]
                                n281 = global write "全局 实时数据参数.vi" "实时数据参数"("水样测试" ("实时数据参数")) -> ()
                                n282 = Get Date/Time In Seconds() -> (seconds since 1Jan1904=w335:timestamp)
                                n283 = Format Date/Time String(time format string (%c)="%Y%m%d%H%M%S%3u" ("时间格式字符串(%c)"), seconds (now)=w335) -> (date/time string=w336:string)  [unwired: 1 in]
                                n284 = Search and Replace String(input string=w336, search string="." ("搜索字符串")) -> (result string=w338:string)  [unwired: 6 in, 3 out]
                                n285 = local read "MN"() -> (w330:string)
                                n286 = local read "PW"() -> (w329:string)
                                n287 = local read "数据发送通道"() -> (w328:enum16{"TCP", "VISA"})
                                n288 = call "数据编码.vi"("table输入"="小时数据" ("新元素/子数组"), "QN"=w338, "MN"=w330, "PW"=w329) -> ("通讯包字符串"=w340:string)  [unwired: 10 in, 1 out]
                                n289 = Build Array(w340) -> (w332:string[])
                                n290 = local write "发送报文显示"(w340) -> ()
                                n291 = call "VISATCP组合选择发送.vi"("数据发送通道"=w328, "命令"="write", "写入缓冲区"=w340) -> ()  [unwired: 9 in, 4 out]
                                n292 = call "发送数据记录到文档(子VI).vi"("数组"=w332) -> ()  [unwired: 9 in, 1 out]
                                n293 = local read "判断数据反馈"() -> (w326:bool)
                                n294 = case shown="真" w326 {
                                tunnel: [_ w364] -> w339
                                tunnel: w340 -> [_ w363]
                                tunnel: w342 -> [_ w362]
                                frame False {
                                }
                                frame True {
                                n295 = case shown="0, 默认" w362 {
                                tunnel: [w366 _] -> w364
                                tunnel: w363 -> [w365 _]
                                frame 0, Default {
                                n296 = Empty String/Path?(string/path=w365) -> (empty?=w367:bool)
                                n297 = case shown="假" w367 {
                                tunnel: [w370 _] -> w366
                                tunnel: w365 -> [w369 _]
                                frame False {
                                n298 = local read "数据发送通道"() -> (w368:enum16{"TCP", "VISA"})
                                n299 = call "数据补发判定有限循环.vi"("数据输入"=w369, "数据发送通道"=w368) -> ("error out"=w370:errorcluster)  [unwired: 9 in]
                                }
                                frame True {
                                }
                                }
                                }
                                frame 14..17 {
                                }
                                }
                                }
                                }
                                n300 = local read "2011发送"() -> (w325:bool)
                                n301 = case shown="真" w325 {
                                tunnel: w341 -> [_ w355]
                                tunnel: w339 -> [_ w354]
                                frame False {
                                }
                                frame True {
                                n302 = local read "MN"() -> (w349:string)
                                n303 = local read "PW"() -> (w348:string)
                                n304 = global write "全局 实时数据参数.vi" "实时数据参数"("水样测试" ("实时数据参数")) -> ()
                                n305 = call "数据编码.vi"("table输入"="实时数据" ("新元素/子数组"), "错误常量 2"=w354, "MN"=w349, "PW"=w348) -> ("通讯包字符串"=w353:string)  [unwired: 10 in, 1 out]
                                n306 = Build Array(w353) -> (w351:string[])
                                n307 = local read "数据发送通道"() -> (w347:enum16{"TCP", "VISA"})
                                n308 = local write "发送报文显示"(w353) -> ()
                                n309 = call "发送数据记录到文档(子VI).vi"("数组"=w351) -> ()  [unwired: 9 in, 1 out]
                                n310 = call "VISATCP组合选择发送.vi"("数据发送通道"=w347, "命令"="write", "写入缓冲区"=w353) -> ("错误输出"=w352:errorcluster)  [unwired: 9 in, 3 out]
                                n311 = local read "判断数据反馈"() -> (w344:bool)
                                n312 = case shown="真" w344 {
                                tunnel: w353 -> [_ w358]
                                tunnel: w352 -> [_ w357]
                                tunnel: w355 -> [_ w356]
                                frame False {
                                }
                                frame True {
                                n313 = case shown="0, 默认" w356 {
                                tunnel: w358 -> [w361 _]
                                tunnel: w357 -> [w360 _]
                                frame 0, Default {
                                n314 = local read "数据发送通道"() -> (w359:enum16{"TCP", "VISA"})
                                n315 = call "数据补发判定有限循环.vi"("错误输入（无错误）"=w360, "数据输入"=w361, "数据发送通道"=w359) -> ()  [unwired: 8 in, 1 out]
                                }
                                frame 14..17 {
                                }
                                }
                                }
                                }
                                }
                                }
                              }
                            }
                          }
                        }
                        frame #2 {
                          n316 = global read "全局 数据发送重叠.vi" "数据接收超时指示灯"() -> (w371:bool)
                          n317 = Not(x=w371) -> (.not. x?=w372:bool)
                          n318 = Compound Arithmetic op=AND ("复合运算")(w372, w374) -> (w373:bool)
                          n319 = case shown="真" w373 {
                            tunnel: w376 -> [_ w380]
                            tunnel: w375 -> [_ w390]
                            tunnel: w377 -> [_ w381]
                            frame False {
                            }
                            frame True {
                              n320 = call "日期时间字符串转换分钟数加一.vi"("data[0]"=w380) -> ("日期/时间字符串"=w378:string)  [unwired: 10 in]
                              n321 = call "时间日期字符串至时间标识转换.vi"("时间日期字符串"=w378) -> ("时间标识"=w379:timestamp)  [unwired: 10 in]
                              n322 = call <vilib>:"Application Directory.vi"() -> ("Application Directory"=w382:path)
                              n323 = case shown="3" w390 {
                                tunnel: w378 -> [w391 w392 w393 w394 w395 w396 w397 w398 w399 w400 w401 w402 w403 w404 w405 w406 w407 w408]
                                frame 0, Default {
                                n324 = global write "全局 水样时间.vi" "time1"(w391) -> ()
                                }
                                frame 1 {
                                n325 = global write "全局 水样时间.vi" "time2"(w392) -> ()
                                }
                                frame 2 {
                                n326 = global write "全局 水样时间.vi" "time3"(w393) -> ()
                                }
                                frame 3 {
                                n327 = global write "全局 水样时间.vi" "time4"(w394) -> ()
                                }
                                frame 4 {
                                n328 = global write "全局 水样时间.vi" "time5"(w395) -> ()
                                }
                                frame 5 {
                                n329 = global write "全局 水样时间.vi" "time6"(w396) -> ()
                                }
                                frame 6 {
                                n330 = global write "全局 水样时间.vi" "time7"(w397) -> ()
                                }
                                frame 7 {
                                n331 = global write "全局 水样时间.vi" "time8"(w398) -> ()
                                }
                                frame 8 {
                                n332 = global write "全局 水样时间.vi" "time9"(w399) -> ()
                                }
                                frame 9 {
                                n333 = global write "全局 水样时间.vi" "time10"(w400) -> ()
                                }
                                frame 10 {
                                n334 = global write "全局 水样时间.vi" "time11"(w401) -> ()
                                }
                                frame 11 {
                                n335 = global write "全局 水样时间.vi" "time12"(w402) -> ()
                                }
                                frame 12 {
                                n336 = global write "全局 水样时间.vi" "time13"(w403) -> ()
                                }
                                frame 13 {
                                n337 = global write "全局 水样时间.vi" "time14"(w404) -> ()
                                }
                                frame 14 {
                                n338 = global write "全局 水样时间.vi" "time15"(w405) -> ()
                                }
                                frame 15 {
                                n339 = global write "全局 水样时间.vi" "time16"(w406) -> ()
                                }
                                frame 16 {
                                n340 = global write "全局 水样时间.vi" "time17"(w407) -> ()
                                }
                                frame 17 {
                                n341 = global write "全局 水样时间.vi" "time18"(w408) -> ()
                                }
                              }
                              n342 = Build Path(base path=w382, name or relative path="data\\Set.ini" ("名称或相对路径")) -> (appended path=w384:path)
                              n343 = call <vilib>:"Open Config Data.vi"("configuration file path"=w384) -> ("error out"=w386:errorcluster, "refnum"=w385:T8)  [unwired: 8 in, 1 out]
                              n344 = local write "数据发送起始时间"(w379) -> ()
                              n345 = call-poly <vilib>:"Write Key.vi"("section"="线程一数据搜索起始时间", "error in (no error)"=w386, "value"=w378, "key"=w381, "refnum"=w385) -> ("error out"=w388:errorcluster, "refnum out"=w387:T8)  [unwired: 4 in, 1 out]
                              n346 = call <vilib>:"Close Config Data.vi"("error in (no error)"=w388, "refnum"=w387) -> ()  [unwired: 8 in, 2 out]
                            }
                          }
                        }
                      }
                    }
                  }
                }
                "实时小时数据上传" <- w163
              }
              frame #1 {
                w445 = FALSE ("小时数据上传")
                n347 = local write "实时小时数据上传"(w445) -> ()
                n348 = global write "全局 数据发送重叠.vi" "主动上报数据中"(w445) -> ()
              }
            }
          }
          frame True {
            # "数据整点触发，整条发送"
          }
        }
      }
    }
  }
  n349 = while {
    stop <- FALSE stop-if-true
    # "数据整点触发，整条发送；数据自动重发设置"
    n350 = global read "断电保存全局.vi" "数据组合发送"() -> (w448:bool)
    n351 = case shown="真" "每周自动重发" {
      frame False {
      }
      frame True {
        (unwired) T1."00点"
        (unwired) T2."关闭"
        # "自动重发水样数据"
        n352 = Get Date/Time In Seconds() -> (seconds since 1Jan1904=w463:timestamp)
        n353 = Seconds To Date/Time(time stamp (now)=w463) -> (date time rec=w457:T9)  [unwired: 1 in]
        n354 = Unbundle By Name(w457) -> ("天数（周）"=w462:i32, "时"=w452:i32, "分"=w461:i32)
        n355 = Equal To 0?(x=w461) -> (x = 0?=w458:bool)
        n356 = Equal?(x=w462, y="重发日期") -> (x = y?=w460:bool)
        n357 = Equal?(x=w452, y="重发时间") -> (x = y?=w459:bool)
        n358 = Compound Arithmetic op=AND ("复合运算")(w460, w459, w458) -> (w456:bool)
        n359 = call <vilib>:"Boolean Crossing PtByPt.vi"("direction"=enum16{"either", "false-true", "true-false"}."false-true", "input"=w456) -> ("crossing"=w455:bool)  [unwired: 1 in]
        n360 = case shown="真" w455 {
          tunnel: w457 -> [_ w466]
          frame False {
          }
          frame True {
            n361 = local read "参数数值"() -> (w464:T5)
            n362 = Unbundle By Name(w466) -> ("日"=w469:i32)
            n363 = Cluster To Array(cluster=w464) -> (array=w471:bool[])
            n364 = Subtract(x=w469, y=7) -> (x-y=w467:i32)
            n365 = Bundle By Name(cluster=w466, "日"=w467) -> (w470:T9)
            n366 = Date/Time To Seconds(2:w470) -> (0:w465:timestamp)  [unwired: 1 in]
            n367 = for {
              tunnel: w471 -> [_] mode=indexing
              tunnel: w465 -> [w472]
              i -> [w473]
              n368 = Format Date/Time String(time format string (%c)="%Y/%m/%d %H:%M:%S" ("时间格式字符串(%c)"), seconds (now)=w472) -> (date/time string=w474:string)  [unwired: 1 in]
              n369 = case shown="16" w473 {
                tunnel: w474 -> [w476 w477 w478 w479 w480 w481 w482 w483 w484 w485 w486 w487 w488 w489 w490 w491 w492 w493]
                frame 0, Default {
                  n370 = global write "全局 水样时间.vi" "time1"(w476) -> ()
                }
                frame 1 {
                  n371 = global write "全局 水样时间.vi" "time2"(w477) -> ()
                }
                frame 2 {
                  n372 = global write "全局 水样时间.vi" "time3"(w478) -> ()
                }
                frame 3 {
                  n373 = global write "全局 水样时间.vi" "time4"(w479) -> ()
                }
                frame 4 {
                  n374 = global write "全局 水样时间.vi" "time5"(w480) -> ()
                }
                frame 5 {
                  n375 = global write "全局 水样时间.vi" "time6"(w481) -> ()
                }
                frame 6 {
                  n376 = global write "全局 水样时间.vi" "time7"(w482) -> ()
                }
                frame 7 {
                  n377 = global write "全局 水样时间.vi" "time8"(w483) -> ()
                }
                frame 8 {
                  n378 = global write "全局 水样时间.vi" "time9"(w484) -> ()
                }
                frame 9 {
                  n379 = global write "全局 水样时间.vi" "time10"(w485) -> ()
                }
                frame 10 {
                  n380 = global write "全局 水样时间.vi" "time11"(w486) -> ()
                }
                frame 11 {
                  n381 = global write "全局 水样时间.vi" "time12"(w487) -> ()
                }
                frame 12 {
                  n382 = global write "全局 水样时间.vi" "time13"(w488) -> ()
                }
                frame 13 {
                  n383 = global write "全局 水样时间.vi" "time14"(w489) -> ()
                }
                frame 14 {
                  n384 = global write "全局 水样时间.vi" "time15"(w490) -> ()
                }
                frame 15 {
                  n385 = global write "全局 水样时间.vi" "time16"(w491) -> ()
                }
                frame 16 {
                  n386 = global write "全局 水样时间.vi" "time17"(w492) -> ()
                }
                frame 17 {
                  n387 = global write "全局 水样时间.vi" "time18"(w493) -> ()
                }
              }
            }
          }
        }
      }
    }
    n388 = case shown="真" w448 {
      frame False {
      }
      frame True {
        n389 = Get Date/Time In Seconds() -> (seconds since 1Jan1904=w501:timestamp)
        n390 = Seconds To Date/Time(time stamp (now)=w501) -> (date time rec=w502:T9)  [unwired: 1 in]
        n391 = global read "断电保存全局.vi" "数据重发"() -> (w494:bool)
        n392 = Unbundle By Name(w502) -> ("分"=w500:i32)
        n393 = Equal?(x=w500, y=0) -> (x = y?=w498:bool)
        n394 = call <vilib>:"Boolean Crossing PtByPt.vi"("direction"=enum16{"either", "false-true", "true-false"}."false-true", "input"=w498) -> ("crossing"=w496:bool)  [unwired: 1 in]
        n395 = Or(x=w494, y=w496) -> (x .or. y?=w495:bool)
        n396 = case shown="真" w495 {
          frame False {
            n397 = global write "全局 数据发送重叠.vi" "主动上报数据中"(FALSE ("主动上报数据中")) -> ()
          }
          frame True {
            n398 = local read "数据发送通道"() -> (w506:enum16{"TCP", "VISA"})
            n399 = local read "MN"() -> (w505:string)
            n400 = local read "PW"() -> (w504:string)
            n401 = call "数据全参数一起发送整点触发.vi"("数据发送通道"=w506, "PW"=w504, "MN"=w505) -> ()  [unwired: 8 in]
          }
        }
      }
    }
    n402 = Wait (ms)(milliseconds to wait=u32 1000 ("等待时间（毫秒）")) -> ()  [unwired: 1 out]
  }
  n403 = Obtain Queue(name (unnamed)="STEP" ("名称（未命名）"), element data type=T6."初始化" ("枚举")) -> (queue out=w53:refnum<queue>)  [unwired: 3 in, 2 out]
  n404 = Insert Into Array(array=string[] [] ("tables"), index=0 ("索引"), new element="实时数据" ("新元素/子数组")) -> (w56:string[])
  n405 = Enqueue Element(queue=w53, element=T6."初始化" ("元素")) -> (queue out=w58:refnum<queue>)  [unwired: 2 in, 2 out]
  "主队列输出" <- w58
  n406 = Array Size(array=w56) -> (size(s)=w54:i32)
  n407 = while {
    stop <- FALSE stop-if-true
    # "心跳包"
    n408 = local read "数据发送通道"() -> (w514:enum16{"TCP", "VISA"})
    n409 = global read "全局 数据发送重叠.vi" "掉线指示灯"() -> (→"掉线指示":bool)
    n410 = Get Date/Time In Seconds() -> (seconds since 1Jan1904=w554:timestamp)
    n411 = local read "数据发送通道"() -> (w529:enum16{"TCP", "VISA"})
    n412 = local read "空闲时间"() -> (w546:dbl)
    n413 = case shown="\"VISA\"" w514 {
      tunnel: [w586 w589] -> w533
      tunnel: [w585 w587] -> w532
      frame "TCP", Default {
        n414 = local read "PORT"() -> (w585:string)
        n415 = local read "IP"() -> (w586:string)
      }
      frame "VISA" {
        n416 = local read "baud rate"() -> (w588:u32)
        n417 = local read "VISA resource name"() -> (w589:refnum<visa-resource-name>)
        n418 = Number To Decimal String(number=w588) -> (decimal integer string=w587:string)  [unwired: 1 in]
      }
    }
    n419 = Wait (ms)(milliseconds to wait=u32 1000 ("等待时间（毫秒）")) -> ()  [unwired: 1 out]
    n420 = global read "全局 数据发送重叠.vi" "主动上报数据中"() -> (w515:bool)
    n421 = local read "核查数据上传"() -> (w541:bool)
    n422 = local read "空闲时间"() -> (w577:dbl)
    n423 = local read "查询数据发送"() -> (w544:bool)
    n424 = Number To Decimal String(number=w546) -> (decimal integer string=→"空闲时间/s":string)  [unwired: 1 in]
    n425 = local read "站点设备"() -> (w534:string)
    n426 = local read "站点名称"() -> (w535:string)
    n427 = global read "全局 数据发送重叠.vi" "数据接收超时指示灯"() -> (→"数据接收超时指示灯":bool)
    n428 = local read "MN"() -> (w531:string)
    n429 = Format Date/Time String(time format string (%c)="%Y/%m/%d %H:%M:%S" ("时间格式字符串(%c)"), seconds (now)=w554) -> (date/time string=→"系统时间":string)  [unwired: 1 in]
    n430 = local read "PW"() -> (w530:string)
    n431 = local read "步骤"() -> (w571:T6)
    n432 = case shown="\"TCP\", 默认" w529 {
      frame "TCP", Default {
        w590 = TRUE ("可见")
        w591 = FALSE ("可见")
        n433 = property on="VISA resource name" class="VISAName"("Visible"=w591) -> ()  [unwired: 2 in, 2 out]
        n434 = property on="baud rate" class="DigNum (严格)"("Visible"=w591) -> ()  [unwired: 2 in, 2 out]
        n435 = property on="IP" class="Str"("Visible"=w590) -> ()  [unwired: 2 in, 2 out]
        n436 = property on="PORT" class="Str"("Visible"=w590) -> ()  [unwired: 2 in, 2 out]
      }
      frame "VISA" {
        w592 = TRUE ("可见")
        w593 = FALSE ("可见")
        n437 = property on="baud rate" class="DigNum (严格)"("Visible"=w592) -> ()  [unwired: 2 in, 2 out]
        n438 = property on="VISA resource name" class="VISAName"("Visible"=w592) -> ()  [unwired: 2 in, 2 out]
        n439 = property on="IP" class="Str"("Visible"=w593) -> ()  [unwired: 2 in, 2 out]
        n440 = property on="PORT" class="Str"("Visible"=w593) -> ()  [unwired: 2 in, 2 out]
      }
    }
    n441 = local read "数据发送协议"() -> (w527:enum16{"2005-212协议", "2017-212协议"})
    n442 = Not(x=w541) -> (.not. x?=w542:bool)
    n443 = Greater?(x=w577, y=30.0) -> (0:w575:bool)
    n444 = Not(x=w515) -> (.not. x?=w543:bool)
    n445 = property on="数据发送通道" class="Enum (严格)"("Visible"="锁") -> ()  [unwired: 2 in, 2 out]
    n446 = Not(x=w544) -> (.not. x?=w565:bool)
    n447 = Equal?(x=w571, y=T6."读取数据" ("步骤")) -> (x = y?=w569:bool)
    n448 = Bundle By Name(cluster=T4 {"站点"="", "设备"="", "IP"="", "PORT"="", "MN"="", "PW"=""} ("配置信息"), "站点"=w535, "设备"=w534, "IP"=w533, "PORT"=w532, "MN"=w531, "PW"=w530) -> (→"配置信息":T4)
    n449 = Select(t=T10."Enabled" ("禁用"), s="更改起始时间", f=T10."Disabled and Grayed Out" ("禁用")) -> (s? t:f=w557:T10)
    n450 = case shown="真" w575 {
      tunnel: w575 -> [_ w603]
      tunnel: [FALSE w603] -> w572
      frame False {
      }
      frame True {
        n451 = local read "QN"() -> (w601:string)
        n452 = local write "空闲时间"(0.0 ("空闲时间")) -> ()
        n453 = local read "MN"() -> (w600:string)
        n454 = local read "PW"() -> (w599:string)
        n455 = global read "断电保存全局.vi" "数据发送通道"() -> (w595:enum16{"TCP", "VISA"})
        n456 = call "数据编码.vi"("table输入"="心跳包", "QN"=w601, "MN"=w600, "PW"=w599) -> ("通讯包字符串"=w597:string)  [unwired: 10 in, 1 out]
        n457 = local write "发送报文显示"(w597) -> ()
        n458 = call "VISATCP组合选择发送.vi"("数据发送通道"=w595, "命令"="write", "写入缓冲区"=w597) -> ("错误输出"=w596:errorcluster)  [unwired: 9 in, 3 out]
        n459 = call <vilib>:"Clear Errors.vi"("error in (no error)"=w596) -> ()  [unwired: 5 in, 2 out]
      }
    }
    "心跳包" <- w572
    n460 = Select(t=T10."Enabled" ("禁用"), s="锁", f=T10."Disabled and Grayed Out" ("禁用")) -> (s? t:f=w520:T10)
    n461 = property on="数据发送起始时间" class="AbsTime (严格)"("DisabledEnum"=w557) -> ()  [unwired: 2 in, 2 out]
    n462 = global read "全局 时间2.vi" "跨度核查索引起始时间"() -> (→"跨度核查索引起始时间":string)
    n463 = case shown="\"2017-212协议\", 默认" w527 {
      tunnel: ["32" ("设备编码MN") w580] -> w563
      frame "2005-212协议" {
      }
      frame "2017-212协议", Default {
        n464 = local read "系统编码选择框"() -> (w581:string)
        n465 = case shown="\"地表水质量监测\", 默认" w581 {
          tunnel: ["52" ("设备编码MN") "32" ("设备编码MN") "21" ("设备编码MN")] -> w580
          frame "污水排放过程监测" {
          }
          frame "地表水体污染源" {
          }
          frame "地表水质量监测", Default {
          }
        }
      }
    }
    n466 = global read "全局 时间2.vi" "标样核查索引起始时间"() -> (→"标样核查索引起始时间":string)
    n467 = global read "全局 时间2.vi" "零点核查索引起始时间"() -> (→"零点核查索引起始时间":string)
    n468 = global read "全局 时间2.vi" "加标回收索引起始时间"() -> (→"加标回收索引起始时间":string)
    n469 = property on="设置超时时间/min" class="DigNum (严格)"("DisabledEnum"=w520) -> ()  [unwired: 2 in, 2 out]
    n470 = property on="IP" class="Str"("DisabledEnum"=w520) -> ()  [unwired: 2 in, 2 out]
    n471 = property on="每周自动重发" class="Bool (严格)"("DisabledEnum"=w520) -> ()  [unwired: 2 in, 2 out]
    n472 = property on="PORT" class="Str"("DisabledEnum"=w520) -> ()  [unwired: 2 in, 2 out]
    n473 = local read "数据发送协议"() -> (w526:enum16{"2005-212协议", "2017-212协议"})
    n474 = local read "TCP服务端掉线计数"() -> (w549:i32)
    n475 = local read "1st Error to Convert"() -> (w552:i32)
    n476 = local read "TCP掉线时间节点"() -> (w548:string)
    n477 = property on="确定更改起始时间" class="Bool"("DisabledEnum"=w557) -> ()  [unwired: 2 in, 2 out]
    n478 = property on="MN" class="Str"("DisabledEnum"=w520) -> ()  [unwired: 2 in, 2 out]
    n479 = property on="PW" class="Str"("DisabledEnum"=w520) -> ()  [unwired: 2 in, 2 out]
    n480 = local read "元素"() -> (w550:string)
    n481 = local read "步骤"() -> (w551:T6)
    n482 = Equal?(x=w526, y=enum16{"2005-212协议", "2017-212协议"}."2017-212协议" ("数据发送协议")) -> (x = y?=w524:bool)
    n483 = Compound Arithmetic op=AND ("复合运算")(w524, w569, w565, w543, w542) -> (w566:bool)
    n484 = case shown="真" w566 {
      frame False {
      }
      frame True {
        n485 = local read "空闲时间"() -> (w606:dbl)
        n486 = Increment(x=w606) -> (x+1=→"空闲时间":dbl)
      }
    }
    n487 = property on="数据发送通道" class="Enum (严格)"("DisabledEnum"=w520) -> ()  [unwired: 2 in, 2 out]
    n488 = Bundle By Name(cluster=T3 {"1st Error to Convert "=54, "步骤 "=enum."打开连接", "元素"="实时数据", "TCP服务端掉线计数"=4, "TCP掉线时间节点"="2019/05/08 15:24:17"} ("状态信息"), "1st Error to Convert"=w552, "步骤"=w551, "元素"=w550, "TCP服务端掉线计数"=w549, "TCP掉线时间节点"=w548) -> (→"状态信息":T3)
    n489 = global read "全局1.vi" "通讯包字符串"() -> (w516:string)
    n490 = property on="重发时间" class="Enum (严格)"("DisabledEnum"=w520) -> ()  [unwired: 2 in, 2 out]
    n491 = property on="重发日期" class="Enum (严格)"("DisabledEnum"=w520) -> ()  [unwired: 2 in, 2 out]
    n492 = property on="VISA resource name" class="VISAName"("DisabledEnum"=w520) -> ()  [unwired: 2 in, 2 out]
    n493 = property on="判断数据反馈" class="Bool (严格)"("DisabledEnum"=w520) -> ()  [unwired: 2 in, 2 out]
    n494 = property on="baud rate" class="DigNum (严格)"("DisabledEnum"=w520) -> ()  [unwired: 2 in, 2 out]
    n495 = property on="数据发送协议" class="Enum (严格)"("DisabledEnum"=w520) -> ()  [unwired: 2 in, 2 out]
    n496 = property on="2011发送" class="Bool (严格)"("DisabledEnum"=w520) -> ()  [unwired: 2 in, 2 out]
    n497 = feedback #1(w516) -> (w517:string)
    n498 = feedback-in #1(w516) -> ()
    n499 = global write "全局1.vi" "系统编码ST"(w563) -> ()
    n500 = property on="日志、参数发送" class="Bool (严格)"("DisabledEnum"=w520) -> ()  [unwired: 2 in, 2 out]
    n501 = property on="数据组合发送" class="Bool (严格)"("DisabledEnum"=w520) -> ()  [unwired: 2 in, 2 out]
    n502 = Not Equal?(x=w516, y=w517) -> (x != y?=w518:bool)
    n503 = case shown="真" w518 {
      tunnel: w516 -> [_ w578]
      frame False {
      }
      frame True {
        n504 = local write "发送报文显示"(w578) -> ()
      }
    }
    n505 = global read "断电保存全局.vi" "日志、参数发送"() -> (w521:bool)
    n506 = global read "断电保存全局.vi" "数据组合发送"() -> (w519:bool)
    n507 = global read "全局1.vi" "读取报文显示"() -> (w508:string)
    n508 = global read "全局1.vi" "发送报文显示"() -> (w507:string)
    n509 = global read "断电保存全局.vi" "数据发送协议"() -> (w513:enum16{"2005-212协议", "2017-212协议"})
    n510 = global read "断电保存全局.vi" "判断数据反馈"() -> (w523:bool)
    n511 = global read "断电保存全局.vi" "数据发送通道"() -> (w512:enum16{"TCP", "VISA"})
    n512 = global read "断电保存全局.vi" "2011发送"() -> (w522:bool)
    n513 = local read "QN"() -> (w509:string)
    n514 = local write "日志、参数发送"(w521) -> ()
    n515 = local write "数据组合发送"(w519) -> ()
    n516 = local write "读取报文显示"(w508) -> ()
    n517 = local write "数据发送协议"(w513) -> ()
    n518 = local write "判断数据反馈"(w523) -> ()
    n519 = local write "数据发送通道"(w512) -> ()
    n520 = local write "发送报文显示"(w507) -> ()
    n521 = local write "2011发送"(w522) -> ()
    n522 = global write "全局1.vi" "MN"("MN") -> ()
    n523 = global write "全局1.vi" "PW"("PW") -> ()
    n524 = global write "全局1.vi" "QN"(w509) -> ()
  }
  n525 = vi-ref "数据传输系统.lvlib:最小窗口后台运行(子VI).vi"() -> (w38:refnum<vi>)
  n526 = while {
    stop <- FALSE stop-if-true
    # "定期释放缓存"
    n527 = Wait (ms)(milliseconds to wait=u32 600000 ("等待时间（毫秒）")) -> ()  [unwired: 1 out]
    n528 = dll-call lib="PTH2[abs F\tgitkrakenCC0平台数采程序 - V1.0.1（修改迭代版）dataFreeMem.dll" fn="FreeMem"() -> ()  [unwired: 4 in, 2 out]
  }
  n529 = while {
    stop <- FALSE stop-if-true
    n530 = event shown="[6] \"判断数据反馈\", \"2011发送\", \"日志、参数发送\", \"数据组合发送\", \"数据发送通道\", \"数据发送协议\": 值改变" {
      selector: _ -> [_ _ _ _ _ _ _ _ _ _ _ _ _ _ _ _]
      dyn-events: _ -> [_ _ _ _ _ _ _ _ _ _ _ _ _ _ _ _]
      timeout: _ -> [_ _ _ _ _ _ _ _ _ _ _ _ _ _ _ _]
      event Timeout {
        n531 = event-data() -> ()  [unwired: 1 in, 2 out]
      }
      event "站点名称", "站点设备", "IP", "PORT", "MN", "PW", "VISA resource name", "baud rate": Value Change {
        w612 = "线程一自主部署站点保存"
        # "TCP服务器端口掉线"
        n532 = event-data() -> ()  [unwired: 1 in, 6 out]
        n533 = call <vilib>:"Application Directory.vi"() -> ("Application Directory"=w654:path)
        n534 = local read "站点名称"() -> (w633:string)
        n535 = Build Path(base path=w654, name or relative path="data\\Set.ini" ("名称或相对路径")) -> (appended path=w652:path)
        n536 = call <vilib>:"Open Config Data.vi"("configuration file path"=w652) -> ("error out"=w650:errorcluster, "refnum"=w651:T8)  [unwired: 8 in, 1 out]
        n537 = local read "站点设备"() -> (w632:string)
        n538 = call-poly <vilib>:"Write Key.vi"("section"=w612, "error in (no error)"=w650, "value"=w633, "key"="站点名称", "refnum"=w651) -> ("error out"=w647:errorcluster, "refnum out"=w648:T8)  [unwired: 4 in, 1 out]
        n539 = call-poly <vilib>:"Write Key.vi"("section"=w612, "error in (no error)"=w647, "value"=w632, "key"="站点设备", "refnum"=w648) -> ("error out"=w644:errorcluster, "refnum out"=w645:T8)  [unwired: 4 in, 1 out]
        n540 = local read "IP"() -> (w631:string)
        n541 = call-poly <vilib>:"Write Key.vi"("section"=w612, "error in (no error)"=w644, "value"=w631, "key"="IP", "refnum"=w645) -> ("error out"=w642:errorcluster, "refnum out"=w643:T8)  [unwired: 4 in, 1 out]
        n542 = local read "PORT"() -> (w630:string)
        n543 = call-poly <vilib>:"Write Key.vi"("section"=w612, "error in (no error)"=w642, "value"=w630, "key"="PORT", "refnum"=w643) -> ("error out"=w640:errorcluster, "refnum out"=w641:T8)  [unwired: 4 in, 1 out]
        n544 = local read "MN"() -> (w624:string)
        n545 = call-poly <vilib>:"Write Key.vi"("section"=w612, "error in (no error)"=w640, "value"=w624, "key"="MN", "refnum"=w641) -> ("error out"=w625:errorcluster, "refnum out"=w628:T8)  [unwired: 4 in, 1 out]
        n546 = local read "PW"() -> (w626:string)
        n547 = call-poly <vilib>:"Write Key.vi"("section"=w612, "error in (no error)"=w625, "value"=w626, "key"="PW", "refnum"=w628) -> ("error out"=w613:errorcluster, "refnum out"=w614:T8)  [unwired: 4 in, 1 out]
        n548 = local read "VISA resource name"() -> (w620:refnum<visa-resource-name>)
        n549 = local read "主队列输出"() -> (w639:refnum<queue>)
        n550 = call-poly <vilib>:"Write Key.vi"("section"=w612, "error in (no error)"=w613, "value"=w620, "key"="VISA", "refnum"=w614) -> ("error out"=w619:errorcluster, "refnum out"=w616:T8)  [unwired: 4 in, 1 out]
        n551 = local read "baud rate"() -> (w618:u32)
        n552 = Flush Queue(queue=w639) -> (queue out=w638:refnum<queue>)  [unwired: 1 in, 2 out]
        n553 = call-poly <vilib>:"Write Key.vi"("section"=w612, "error in (no error)"=w619, "value"=w618, "key"="BAUDRATE", "refnum"=w616) -> ("error out"=w610:errorcluster, "refnum out"=w611:T8)  [unwired: 4 in, 1 out]
        n554 = local read "数据发送通道"() -> (w623:enum16{"TCP", "VISA"})
        n555 = call <vilib>:"Close Config Data.vi"("error in (no error)"=w610, "refnum"=w611) -> ()  [unwired: 8 in, 2 out]
        n556 = call "VISATCP组合选择发送.vi"("数据发送通道"=w623, "命令"="close") -> ("错误输出"=w621:errorcluster)  [unwired: 10 in, 3 out]
        n557 = Enqueue Element(queue=w638, element=T6."初始化" ("元素"), timeout in ms (-1)=1000 ("超时毫秒(-1)")) -> ()  [unwired: 1 in, 3 out]
        n558 = call <vilib>:"Clear Errors.vi"("error in (no error)"=w621) -> ()  [unwired: 5 in, 2 out]
      }
      event "确定": Value Change {
        w659 = "线程一自主部署站点保存"
        # "TCP服务器端口掉线"
        n559 = event-data() -> ()  [unwired: 1 in, 6 out]
        n560 = call <vilib>:"Application Directory.vi"() -> ("Application Directory"=w692:path)
        n561 = local read "站点名称"() -> (w687:string)
        n562 = Build Path(base path=w692, name or relative path="data\\Set.ini" ("名称或相对路径")) -> (appended path=w690:path)
        n563 = call <vilib>:"Open Config Data.vi"("configuration file path"=w690) -> ("error out"=w688:errorcluster, "refnum"=w689:T8)  [unwired: 8 in, 1 out]
        n564 = local read "站点设备"() -> (w682:string)
        n565 = call-poly <vilib>:"Write Key.vi"("section"=w659, "error in (no error)"=w688, "value"=w687, "key"="站点名称", "refnum"=w689) -> ("error out"=w684:errorcluster, "refnum out"=w685:T8)  [unwired: 4 in, 1 out]
        n566 = call-poly <vilib>:"Write Key.vi"("section"=w659, "error in (no error)"=w684, "value"=w682, "key"="站点设备", "refnum"=w685) -> ("error out"=w680:errorcluster, "refnum out"=w681:T8)  [unwired: 4 in, 1 out]
        n567 = local read "IP"() -> (w675:string)
        n568 = local read "PORT"() -> (w674:string)
        n569 = call-poly <vilib>:"Write Key.vi"("section"=w659, "error in (no error)"=w680, "value"=w675, "key"="IP", "refnum"=w681) -> ("error out"=w678:errorcluster, "refnum out"=w679:T8)  [unwired: 4 in, 1 out]
        n570 = call-poly <vilib>:"Write Key.vi"("section"=w659, "error in (no error)"=w678, "value"=w674, "key"="PORT", "refnum"=w679) -> ("error out"=w670:errorcluster, "refnum out"=w671:T8)  [unwired: 4 in, 1 out]
        n571 = local read "MN"() -> (w667:string)
        n572 = call-poly <vilib>:"Write Key.vi"("section"=w659, "error in (no error)"=w670, "value"=w667, "key"="MN", "refnum"=w671) -> ("error out"=w668:errorcluster, "refnum out"=w669:T8)  [unwired: 4 in, 1 out]
        n573 = local read "PW"() -> (w666:string)
        n574 = call-poly <vilib>:"Write Key.vi"("section"=w659, "error in (no error)"=w668, "value"=w666, "key"="PW", "refnum"=w669) -> ("error out"=w664:errorcluster, "refnum out"=w665:T8)  [unwired: 4 in, 1 out]
        n575 = call <vilib>:"Close Config Data.vi"("error in (no error)"=w664, "refnum"=w665) -> ("error out"=w658:errorcluster)  [unwired: 8 in, 1 out]
        n576 = local read "主队列输出"() -> (w663:refnum<queue>)
        n577 = local read "数据发送通道"() -> (w657:enum16{"TCP", "VISA"})
        n578 = call "VISATCP组合选择发送.vi"("数据发送通道"=w657, "命令"="close") -> ("错误输出"=w655:errorcluster)  [unwired: 10 in, 3 out]
        n579 = Flush Queue(queue=w663) -> (queue out=w662:refnum<queue>)  [unwired: 1 in, 2 out]
        n580 = case shown="错误" w658 {
          frame No Error {
            n581 = One Button Dialog(message="保存成功" ("消息"), button name ("OK")="确定" ("按钮名称（“确定”）")) -> ()  [unwired: 1 out]
          }
          frame Error {
            n582 = One Button Dialog(message="保存失败" ("消息"), button name ("OK")="确定" ("按钮名称（“确定”）")) -> ()  [unwired: 1 out]
          }
        }
        n583 = call <vilib>:"Clear Errors.vi"("error in (no error)"=w655) -> ()  [unwired: 5 in, 2 out]
        n584 = Enqueue Element(queue=w662, element=T6."初始化" ("元素"), timeout in ms (-1)=1000 ("超时毫秒(-1)")) -> ()  [unwired: 1 in, 3 out]
      }
      event "参数配置": Value Change {
        n585 = event-data() -> ()  [unwired: 1 in, 6 out]
        n586 = property on="窗格" class="Pane"("Origin"=T11 {"Horizontal"=0, "Vertical"=1000} ("原点")) -> ()  [unwired: 2 in, 2 out]
      }
      event "返回": Value Change {
        n587 = event-data() -> ()  [unwired: 1 in, 6 out]
        n588 = property on="窗格" class="Pane"("Origin"=T11 {"Horizontal"=0, "Vertical"=0} ("原点")) -> ()  [unwired: 2 in, 2 out]
      }
      event "系统编码选择框": Value Change {
        n589 = event-data() -> ()  [unwired: 1 in, 6 out]
        n590 = call <vilib>:"Application Directory.vi"() -> ("Application Directory"=w707:path)
        n591 = Build Path(base path=w707, name or relative path="data\\Set.ini" ("名称或相对路径")) -> (appended path=w708:path)
        n592 = call <vilib>:"Open Config Data.vi"("configuration file path"=w708) -> ("error out"=w704:errorcluster, "refnum"=w705:T8)  [unwired: 8 in, 1 out]
        n593 = call-poly <vilib>:"Write Key.vi"("section"="系统编码选择", "error in (no error)"=w704, "value"="系统编码选择框", "key"="系统编码", "refnum"=w705) -> ("error out"=w702:errorcluster, "refnum out"=w703:T8)  [unwired: 4 in, 1 out]
        n594 = call <vilib>:"Close Config Data.vi"("error in (no error)"=w702, "refnum"=w703) -> ()  [unwired: 8 in, 2 out]
      }
      event "判断数据反馈", "2011发送", "日志、参数发送", "数据组合发送", "数据发送通道", "数据发送协议": Value Change {
        n595 = event-data() -> ()  [unwired: 1 in, 6 out]
        n596 = flat-sequence {
          frame #0 {
            n597 = global write "断电保存全局.vi" "日志、参数发送"("日志、参数发送") -> ()
            n598 = global write "断电保存全局.vi" "判断数据反馈"("判断数据反馈") -> ()
            n599 = global write "断电保存全局.vi" "数据发送通道"("数据发送通道") -> ()
            n600 = global write "断电保存全局.vi" "2011发送"("2011发送") -> ()
            n601 = global write "断电保存全局.vi" "数据组合发送"("数据组合发送") -> ()
            n602 = global write "断电保存全局.vi" "数据发送协议"("数据发送协议") -> ()
          }
          frame #1 {
            n603 = call <vilib>:"Application Directory.vi"() -> ("Application Directory"=w715:path)
            n604 = Build Path(base path=w715, name or relative path="data\\sys.ini" ("名称或相对路径")) -> (appended path=w717:path)
            n605 = call <vilib>:"Open Config Data.vi"("configuration file path"=w717) -> ("error out"=w721:errorcluster, "refnum"=w718:T8)  [unwired: 8 in, 1 out]
            n606 = vi-ref "断电保存全局.vi"() -> (w719:refnum<vi>)
            n607 = call <userlib>:"Write Panel to INI__ogtk.vi"("error in (no error)"=w721, "VI ref"=w719, "refnum"=w718) -> ("error out"=w722:errorcluster, "refnum out"=w720:T8)  [unwired: 7 in]
            n608 = call <vilib>:"Close Config Data.vi"("error in (no error)"=w722, "refnum"=w720) -> ("error out"=w727:errorcluster, "file path"=w728:path)  [unwired: 8 in]
            n609 = Open/Create/Replace File(file path (use dialog)=w728, error in=w727) -> (refnum out=w724:refnum<file>, error out=w723:errorcluster)  [unwired: 4 in, 1 out]
            n610 = Flush File(refnum=w724, error in=w723) -> (refnum out=w725:refnum<file>, error out=w726:errorcluster)
            n611 = Close File(refnum=w725, error in=w726) -> ()  [unwired: 2 out]
          }
        }
      }
      event "每周自动重发": Value Change {
        n612 = event-data() -> ()  [unwired: 1 in, 6 out]
        n613 = call <vilib>:"Application Directory.vi"() -> ("Application Directory"=w737:path)
        n614 = Build Path(base path=w737, name or relative path="data\\Set.ini" ("名称或相对路径")) -> (appended path=w738:path)
        n615 = local read "每周自动重发"() -> (w729:bool)
        n616 = call <vilib>:"Open Config Data.vi"("configuration file path"=w738) -> ("error out"=w734:errorcluster, "refnum"=w735:T8)  [unwired: 8 in, 1 out]
        n617 = call-poly <vilib>:"Write Key.vi"("section"="线程一数据重发功能", "error in (no error)"=w734, "value"=w729, "key"="重发功能", "refnum"=w735) -> ("error out"=w732:errorcluster, "refnum out"=w733:T8)  [unwired: 4 in, 1 out]
        n618 = call <vilib>:"Close Config Data.vi"("error in (no error)"=w732, "refnum"=w733) -> ()  [unwired: 8 in, 2 out]
      }
      event "重发日期": Value Change {
        n619 = event-data() -> ()  [unwired: 1 in, 6 out]
        n620 = call <vilib>:"Application Directory.vi"() -> ("Application Directory"=w747:path)
        n621 = Build Path(base path=w747, name or relative path="data\\Set.ini" ("名称或相对路径")) -> (appended path=w748:path)
        n622 = local read "重发日期"() -> (w739:T2)
        n623 = call <vilib>:"Open Config Data.vi"("configuration file path"=w748) -> ("error out"=w744:errorcluster, "refnum"=w745:T8)  [unwired: 8 in, 1 out]
        n624 = call-poly <vilib>:"Write Key.vi"("section"="线程一数据重发功能", "error in (no error)"=w744, "value"=w739, "key"="重发日期", "refnum"=w745) -> ("error out"=w742:errorcluster, "refnum out"=w743:T8)  [unwired: 4 in, 1 out]
        n625 = call <vilib>:"Close Config Data.vi"("error in (no error)"=w742, "refnum"=w743) -> ()  [unwired: 8 in, 2 out]
      }
      event "重发时间": Value Change {
        n626 = event-data() -> ()  [unwired: 1 in, 6 out]
        n627 = call <vilib>:"Application Directory.vi"() -> ("Application Directory"=w757:path)
        n628 = Build Path(base path=w757, name or relative path="data\\Set.ini" ("名称或相对路径")) -> (appended path=w758:path)
        n629 = local read "重发时间"() -> (w749:T1)
        n630 = call <vilib>:"Open Config Data.vi"("configuration file path"=w758) -> ("error out"=w754:errorcluster, "refnum"=w755:T8)  [unwired: 8 in, 1 out]
        n631 = call-poly <vilib>:"Write Key.vi"("section"="线程一数据重发功能", "error in (no error)"=w754, "value"=w749, "key"="重发时间", "refnum"=w755) -> ("error out"=w752:errorcluster, "refnum out"=w753:T8)  [unwired: 4 in, 1 out]
        n632 = call <vilib>:"Close Config Data.vi"("error in (no error)"=w752, "refnum"=w753) -> ()  [unwired: 8 in, 2 out]
      }
      event "确定更改起始时间": Value Change {
        n633 = event-data() -> ()  [unwired: 1 in, 6 out]
        n634 = local write "更改起始时间"(FALSE ("更改起始时间")) -> ()
        n635 = Two Button Dialog(message="确定以当前设置时间作为数据索引起始时间？" ("消息")) -> (T button?=w760:bool)  [unwired: 2 in]
        n636 = case shown="真" w760 {
          frame False {
          }
          frame True {
            n637 = local read "参数数值"() -> (w765:T5)
            n638 = global write "断电保存全局.vi" "数据重发"(TRUE ("数据重发")) -> ()
            n639 = Cluster To Array(cluster=w765) -> (array=w766:bool[])
            n640 = for {
              tunnel: w766 -> [_] mode=indexing
              tunnel: [w776] -> w764
              i -> [w777]
              n641 = Format Date/Time String(time format string (%c)="%Y/%m/%d %H:%M:%S" ("时间格式字符串(%c)"), seconds (now)="数据发送起始时间") -> (date/time string=w776:string)  [unwired: 1 in]
              n642 = global write "断电保存全局.vi" "数据重发时间戳"(w776) -> ()
              n643 = case shown="0, 默认" w777 {
                tunnel: w776 -> [w780 w781 w782 w783 w784 w785 w786 w787 w788 w789 w790 w791 w792 w793 w794 w795 w796 w797]
                frame 0, Default {
                  n644 = global write "全局 水样时间.vi" "time1"(w780) -> ()
                }
                frame 1 {
                  n645 = global write "全局 水样时间.vi" "time2"(w781) -> ()
                }
                frame 2 {
                  n646 = global write "全局 水样时间.vi" "time3"(w782) -> ()
                }
                frame 3 {
                  n647 = global write "全局 水样时间.vi" "time4"(w783) -> ()
                }
                frame 4 {
                  n648 = global write "全局 水样时间.vi" "time5"(w784) -> ()
                }
                frame 5 {
                  n649 = global write "全局 水样时间.vi" "time6"(w785) -> ()
                }
                frame 6 {
                  n650 = global write "全局 水样时间.vi" "time7"(w786) -> ()
                }
                frame 7 {
                  n651 = global write "全局 水样时间.vi" "time8"(w787) -> ()
                }
                frame 8 {
                  n652 = global write "全局 水样时间.vi" "time9"(w788) -> ()
                }
                frame 9 {
                  n653 = global write "全局 水样时间.vi" "time10"(w789) -> ()
                }
                frame 10 {
                  n654 = global write "全局 水样时间.vi" "time11"(w790) -> ()
                }
                frame 11 {
                  n655 = global write "全局 水样时间.vi" "time12"(w791) -> ()
                }
                frame 12 {
                  n656 = global write "全局 水样时间.vi" "time13"(w792) -> ()
                }
                frame 13 {
                  n657 = global write "全局 水样时间.vi" "time14"(w793) -> ()
                }
                frame 14 {
                  n658 = global write "全局 水样时间.vi" "time15"(w794) -> ()
                }
                frame 15 {
                  n659 = global write "全局 水样时间.vi" "time16"(w795) -> ()
                }
                frame 16 {
                  n660 = global write "全局 水样时间.vi" "time17"(w796) -> ()
                }
                frame 17 {
                  n661 = global write "全局 水样时间.vi" "time18"(w797) -> ()
                }
              }
            }
            n662 = global read "断电保存全局.vi" "数据组合发送"() -> (w762:bool)
            n663 = case shown="假" w762 {
              tunnel: w764 -> [w767 _]
              frame False {
                n664 = global write "全局 时间2.vi" "跨度核查索引起始时间"(w767) -> ()
                n665 = global write "全局 时间2.vi" "标样核查索引起始时间"(w767) -> ()
                n666 = global write "全局 时间2.vi" "零点核查索引起始时间"(w767) -> ()
                n667 = global write "全局 时间2.vi" "加标回收索引起始时间"(w767) -> ()
                n668 = for {
                  N: 5 -> [_]
                  tunnel: w767 -> [w769]
                  i -> [w770]
                  n669 = case shown="4" w770 {
                    tunnel: w769 -> [w771 w772 w773 w774 w775]
                    frame 0, Default {
                      n670 = global write "全局 时间2.vi" "氨氮跨度核查索引起始时间"(w771) -> ()
                      n671 = global write "全局 时间2.vi" "氨氮零点核查索引起始时间"(w771) -> ()
                    }
                    frame 1 {
                      n672 = global write "全局 时间2.vi" "总氮跨度核查索引起始时间"(w772) -> ()
                      n673 = global write "全局 时间2.vi" "总氮零点核查索引起始时间"(w772) -> ()
                    }
                    frame 2 {
                      n674 = global write "全局 时间2.vi" "总磷跨度核查索引起始时间"(w773) -> ()
                      n675 = global write "全局 时间2.vi" "总磷零点核查索引起始时间"(w773) -> ()
                    }
                    frame 3 {
                      n676 = global write "全局 时间2.vi" "CODMn跨度核查索引起始时间"(w774) -> ()
                      n677 = global write "全局 时间2.vi" "CODMn零点核查索引起始时间"(w774) -> ()
                    }
                    frame 4 {
                      n678 = global write "全局 时间2.vi" "CODCr跨度核查索引起始时间"(w775) -> ()
                      n679 = global write "全局 时间2.vi" "CODCr零点核查索引起始时间"(w775) -> ()
                    }
                  }
                }
              }
              frame True {
              }
            }
          }
        }
      }
      event "开机启动": Value Change {
        n680 = event-data() -> ("NewVal"=w798:bool)  [unwired: 1 in, 5 out]
        n681 = case shown="假" w798 {
          frame False {
            n682 = Two Button Dialog(message="是否删除开机启动" ("消息"), 1:"否" ("F按钮名称（“取消”）"), 2:"是" ("T按钮名称（“确定”）")) -> (T button?=w799:bool)
            n683 = case shown="真" w799 {
              frame False {
              }
              frame True {
                n684 = call <vilib>:"Application Directory.vi"() -> ("Application Directory"=w804:path)
                n685 = call "删除启动项.vi"("启动文件路径"=w804) -> ("删除标记"=w803:bool)  [unwired: 9 in, 1 out]
                n686 = case shown="假" w803 {
                  tunnel: ["删除开机启动失败" ("T按钮名称（“确定”）") "删除开机启动成功" ("T按钮名称（“确定”）")] -> w805
                  frame False {
                  }
                  frame True {
                  }
                }
                n687 = One Button Dialog(message=w805) -> ()  [unwired: 1 in, 1 out]
              }
            }
          }
          frame True {
            n688 = Two Button Dialog(message="是否添加开机启动" ("消息"), 1:"否" ("F按钮名称（“取消”）"), 2:"是" ("T按钮名称（“确定”）")) -> (T button?=w808:bool)
            n689 = case shown="真" w808 {
              frame False {
              }
              frame True {
                n690 = call <vilib>:"Application Directory.vi"() -> ("Application Directory"=w814:path)
                n691 = call "添加启动项.vi"("启动文件路径"=w814) -> ("添加成功标记"=w813:bool)  [unwired: 9 in, 1 out]
                n692 = case shown="真" w813 {
                  tunnel: ["添加开机启动失败" ("T按钮名称（“确定”）") "添加开机启动成功" ("T按钮名称（“确定”）")] -> w812
                  frame False {
                  }
                  frame True {
                  }
                }
                n693 = One Button Dialog(message=w812) -> ()  [unwired: 1 in, 1 out]
              }
            }
          }
        }
      }
      event "IP": Mouse Down {
        n694 = event-data() -> ("CtlRef"=w817:refnum<vi>)  [unwired: 1 in, 5 out]
        n695 = property class="Str" props=["Value"](reference=w817) -> ()  [unwired: 1 in, 3 out]
        n696 = local read "IP"() -> (w819:string)
        n697 = call "IP键盘.vi"("OldNumber"=w819) -> ("NewNumber"=w818:string)
        n698 = local write "IP"(w818) -> ()
      }
      event "PORT": Mouse Down {
        n699 = event-data() -> ()  [unwired: 1 in, 6 out]
        n700 = local read "PORT"() -> (w821:string)
        n701 = call "IP键盘.vi"("OldNumber"=w821) -> ("NewNumber"=w820:string)
        n702 = local write "PORT"(w820) -> ()
      }
      event "查询质控数据起始时间": Value Change {
        n703 = event-data() -> ()  [unwired: 1 in, 6 out]
        n704 = property on="窗格" class="Pane"("Origin"=T11 {"Horizontal"=1000, "Vertical"=0} ("原点")) -> ()  [unwired: 2 in, 2 out]
      }
      event "返回主界面": Value Change {
        n705 = event-data() -> ()  [unwired: 1 in, 6 out]
        n706 = property on="窗格" class="Pane"("Origin"=T11 {"Horizontal"=0, "Vertical"=0} ("原点")) -> ()  [unwired: 2 in, 2 out]
      }
    }
  }
  n707 = while {
    shift-right: [w824] -> _
    shift-left: errorcluster {"status"=FALSE, "code"=0, "source"=""} ("error out") -> [w836]
    shift-right: [w833] -> _
    shift-left: _ -> [w832]
    tunnel: w58 -> [w835]
    tunnel: w56 -> [w831]
    shift-right: [w829] -> _
    shift-left: w36 -> [w830]
    tunnel: w54 -> [w828]
    shift-right: [w826] -> _
    shift-left: w36 -> [w827]
    stop <- FALSE stop-if-true
    n708 = case shown="无错误" w836 {
      selector: w836 -> [w854 w1027]
      tunnel: [w837 w1030] -> w824
      tunnel: w835 -> [w853 w1025]
      tunnel: [w838 w1029] -> w833
      tunnel: w832 -> [w850 w1029]
      tunnel: w831 -> [w849 _]
      tunnel: w830 -> [w844 w1028]
      tunnel: [w847 w1028] -> w829
      tunnel: w828 -> [w846 _]
      tunnel: w827 -> [w841 w1024]
      tunnel: [w840 w1024] -> w826
      frame No Error {
        n709 = Less?(x=w844, y=w846) -> (x < y?=w845:bool)
        n710 = Dequeue Element(queue=w853) -> (queue out=w851:refnum<queue>, element=w852:T6)  [unwired: 2 in, 2 out]
        "步骤" <- w852
        n711 = Select(t=w844, s=w845, f=0) -> (s? t:f=w843:i32)
        n712 = local read "元素"() -> (w839:string)
        n713 = Index Array(array=w849, index=w843) -> (element=→"元素":string)
        n714 = case shown="\"读取数据\"" w852 {
          tunnel: w854 -> [w861 _ w884 w892 w939 w1021]
          tunnel: w851 -> [w858 w875 w879 w906 w937 w1019]
          tunnel: [w861 w863 w884 w890 w936 w1021] -> w837
          tunnel: [string[] [] ("待发送第一条数据") w877 _ w919 w940 _] -> w838
          tunnel: w850 -> [_ w877 _ w919 w940 w1020]
          tunnel: w839 -> [_ _ _ _ _ w1014]
          tunnel: w843 -> [w859 w874 w883 w920 w941 w1010]
          tunnel: [w859 w874 w882 w920 w941 w1011] -> w847
          tunnel: w841 -> [w856 w872 w881 _ w932 w1008]
          tunnel: [w856 w872 w881 0 ("索引") w935 w1008] -> w840
          frame "初始化", Default {
            n715 = Enqueue Element(queue=w858, element=T6."打开连接" ("元素"), timeout in ms (-1)=1000 ("超时毫秒(-1)")) -> ()  [unwired: 1 in, 3 out]
          }
          frame "打开连接" {
            (unwired) "47.98.43.76"
            # "和时通数据接入平台端接收IP端口号，61.191.22.195:10003。"
            # "47.98.43.76:6666"
            n716 = Enqueue Element(queue=w875, element=T6."表格比对" ("元素"), timeout in ms (-1)=1000 ("超时毫秒(-1)")) -> ()  [unwired: 1 in, 3 out]
            n717 = local read "数据发送通道"() -> (w862:enum16{"TCP", "VISA"})
            n718 = call "VISATCP组合选择发送.vi"("IP"="IP", "数据发送通道"=w862, "命令"="open", "PORT"="PORT", "VISA resource name"="VISA resource name", "baud rate"="baud rate") -> ("错误输出"=w863:errorcluster)  [unwired: 6 in, 3 out]
            n719 = Unbundle By Name(w863) -> ("status"=w871:bool, "code"=→"1st Error to Convert":i32)
            n720 = Not(x=w871) -> (.not. x?=→"通信状态":bool)
          }
          frame "表格比对" {
            n721 = Enqueue Element(queue=w879, element=T6."读取数据" ("元素"), timeout in ms (-1)=1000 ("超时毫秒(-1)")) -> ()  [unwired: 1 in, 3 out]
            n722 = Increment(x=w883) -> (x+1=w882:i32)
          }
          frame "读取数据" {
            # "设置测量时间间隔"
            # "1000设置超时时间和重发次数\n1011提取监测仪表时间\n1012设置监测仪表时间\n1014提取数采仪时间\n1015设置数采仪时间\n1061提取实时数据间隔\n1062设置实时数据间隔\n1072设置数采仪访问密码"
            # "6分钟掉线重连"
            n723 = local write "查询数据发送"(FALSE ("数据正在发送")) -> ()
            n724 = global write "全局 数据发送重叠.vi" "掉线指示灯"(FALSE ("数据发送重叠")) -> ()
            n725 = property on="TCP服务端掉线计数" class="DigNum (严格)"("Value"=0 ("TCP服务端掉线计数")) -> ()  [unwired: 2 in, 2 out]
            n726 = local read "数据发送通道"() -> (w894:enum16{"TCP", "VISA"})
            n727 = call "VISATCP组合选择发送.vi"("数据发送通道"=w894, "命令"="read", "error in (no error)"=w892) -> ("读取缓冲区"=w891:string, "错误输出"=w890:errorcluster)  [unwired: 9 in, 2 out]
            n728 = call "读取数据处理 (子VI).vi"("data out"=w891) -> ("系统编码ST"=→"系统编码ST":string, "命令编码CN"=w907:string, "设备编码MN"=→"设备编码MN":string, "密码PW"=→"密码PW":string, "数据"=w888:string, "拆分包及应答Flag"=→"拆分包及应答Flag":string, "时间QN"=w910:string)  [unwired: 6 in, 2 out]
            "命令编码CN" <- w907
            "数据" <- w888
            "时间QN" <- w910
            n729 = Empty String/Path?(string/path=w891) -> (empty?=w900:bool)
            n730 = local read "实时小时数据上传"() -> (w899:bool)
            n731 = case shown="假" w900 {
              tunnel: w891 -> [w927 _]
              frame False {
                n732 = global write "全局1.vi" "数据输出"(w927) -> ()
                n733 = call "数据记录.vi"("写入字段"=w927) -> ("连接的字符串"=→"读取报文显示":string)  [unwired: 10 in]
                "数据输出" <- w927
              }
              frame True {
              }
            }
            n734 = local read "核查数据上传"() -> (w898:bool)
            n735 = Not(x=w899) -> (.not. x?=w897:bool)
            n736 = Not(x=w898) -> (.not. x?=w896:bool)
            n737 = And(x=w897, y=w896) -> (x .and. y?=w895:bool)
            n738 = Search/Split String(string=w910, search string/char (-)="QN=" ("搜索字符串/字符(-)")) -> (match + rest of string=w908:string)  [unwired: 1 in, 2 out]
            n739 = case shown="真" w895 {
              tunnel: w907 -> [_ w925]
              tunnel: ["" ("命令编码CN") w922] -> w901
              frame False {
              }
              frame True {
                n740 = Search/Split String(string=w925, search string/char (-)="CN=" ("搜索字符串/字符(-)")) -> (match + rest of string=w923:string)  [unwired: 1 in, 2 out]
                n741 = String Subset(string=w923, offset (0)=3 ("偏移量(0)")) -> (substring=w922:string)  [unwired: 1 in]
              }
            }
            n742 = String Subset(string=w908, offset (0)=3 ("偏移量(0)")) -> (substring=→"QN":string)  [unwired: 1 in]
            n743 = call "读取数据解析(子VI).vi"("数据"=w888, "命令编码CN"=w901, "队列输入"=w906) -> ("实时数据发送时间间隔/min"=w885:i32, "元素"=w903:T6, "设置超时时间/min"=→"设置超时时间/min":i32, "队列输出"=w904:refnum<queue>, "table"=w886:string)  [unwired: 4 in]
            n744 = local write "table元素"(w886) -> ()
            n745 = global write "实时数据发送间隔全局.vi" "实时数据发送间隔"(w885) -> ()
            n746 = local write "实时数据发送时间间隔/min"(w885) -> ()
            n747 = Enqueue Element(queue=w904, element=w903, timeout in ms (-1)=1000 ("超时毫秒(-1)")) -> ()  [unwired: 1 in, 3 out]
          }
          frame "发送数据" {
            # "table输入，选择命令编码、发送哪些数据"
            n748 = local read "table元素"() -> (w933:string)
            n749 = case shown="\"报警信息\", \"操作日志\", \"核查数据\", \"空白测试\", \"跨度核查\", \"零点核查\", \"实时数据\", \"提取集成干预\", \"提取加标回收\", \"提取平行样\", \"提取实时数据\", \"提取小时数据\", \"提取仪器参数\", \"仪器参数\"" w933 {
              tunnel: w932 -> [w944 w948 w950 w957]
              tunnel: [w942 w947 w951 w955] -> w930
              tunnel: [w943 w946 w952 w956] -> w931
              frame "", Default {
                n750 = global write "全局1.vi" "枚举"(w944) -> ()
                n751 = Increment(x=w944) -> (x+1=w943:i32)
                n752 = Greater Or Equal?(x=w943, y=3) -> (x >= y?=w942:bool)
              }
              frame "反控命令" {
                n753 = global write "全局 反控命令枚举.vi" "反控命令枚举"(w948) -> ()
                n754 = Increment(x=w948) -> (x+1=w946:i32)
                n755 = Greater Or Equal?(x=w946, y=2) -> (x >= y?=w947:bool)
              }
              frame "超标留样返回", "提取监测仪表时间", "提取经纬度环境信息", "提取现场系统信息" {
                n756 = global write "全局1.vi" "枚举"(w950) -> ()
                n757 = Increment(x=w950) -> (x+1=w952:i32)
                n758 = Greater Or Equal?(x=w952, y=3) -> (x >= y?=w951:bool)
              }
              frame "报警信息", "操作日志", "核查数据", "空白测试", "跨度核查", "零点核查", "实时数据", "提取集成干预", "提取加标回收", "提取平行样", "提取实时数据", "提取小时数据", "提取仪器参数", "仪器参数" {
                n759 = global read "全局 小时数据发送次数.vi" "小时数据发送次数"() -> (w959:i32)
                n760 = global read "全局 数据数组大小.vi" "数据数组大小"() -> (w954:i32)
                n761 = Greater Or Equal?(x=w959, y=w954) -> (x >= y?=w960:bool)
                n762 = case shown="真" w960 {
                  tunnel: w957 -> [w965 w972]
                  tunnel: [w965 w966] -> w961
                  frame False {
                  }
                  frame True {
                    n763 = global read "全局 小时数据发送次数.vi" "小时数据发送次数"() -> (w971:i32)
                    n764 = global read "全局 数据数组大小.vi" "数据数组大小"() -> (w968:i32)
                    n765 = Equal To 0?(x=w971) -> (x = 0?=w970:bool)
                    n766 = Equal To 0?(x=w968) -> (x = 0?=w969:bool)
                    n767 = And(x=w970, y=w969) -> (x .and. y?=w967:bool)
                    n768 = case shown="真" w967 {
                      tunnel: w972 -> [w974 _]
                      tunnel: [w973 0 ("索引")] -> w966
                      frame False {
                        n769 = Increment(x=w974) -> (x+1=w973:i32)
                      }
                      frame True {
                      }
                    }
                  }
                }
                n770 = global write "全局1.vi" "枚举"(w961) -> ()
                n771 = Equal To 0?(x=w961) -> (x = 0?=w962:bool)
                n772 = case shown="真" w962 {
                  tunnel: w961 -> [w963 _]
                  tunnel: [w963 1] -> w956
                  frame False {
                  }
                  frame True {
                  }
                }
                n773 = Greater Or Equal?(x=w956, y=2) -> (x >= y?=w955:bool)
              }
            }
            n774 = flat-sequence {
              tunnel: "table元素" -> [w987]
              tunnel: w939 -> [w986]
              tunnel: [w982] -> w938
              tunnel: [w991] -> w936
              tunnel: w938 -> [w991]
              tunnel: w937 -> [w990]
              tunnel: w930 -> [w989]
              frame #0 {
                # "数据记录"
                # "数据编码"
                n775 = local read "MN"() -> (w979:string)
                n776 = local read "QN"() -> (w985:string)
                n777 = local read "PW"() -> (w978:string)
                n778 = call "数据编码.vi"("table输入"=w987, "错误常量 2"=w986, "QN"=w985, "MN"=w979, "PW"=w978) -> ("错误常量"=w984:errorcluster, "通讯包字符串"=w983:string)  [unwired: 9 in]
                n779 = local read "数据发送通道"() -> (w981:enum16{"TCP", "VISA"})
                n780 = call "数据记录.vi"("写入字段"=w983) -> ("连接的字符串"=→"发送报文显示":string)  [unwired: 10 in]
                n781 = call "VISATCP组合选择发送.vi"("数据发送通道"=w981, "命令"="write", "error in (no error)"=w984, "写入缓冲区"=w983) -> ("错误输出"=w982:errorcluster)  [unwired: 8 in, 3 out]
              }
              frame #1 {
                n782 = case shown="真" w989 {
                  tunnel: w990 -> [w992 w1004]
                  frame False {
                    n783 = Enqueue Element(queue=w992, element=T6."发送数据" ("元素")) -> ()  [unwired: 2 in, 3 out]
                  }
                  frame True {
                    n784 = local read "TCP服务端掉线计数"() -> (w999:i32)
                    n785 = Obtain Queue(name (unnamed)="重发掉线数据" ("名称（未命名）"), element data type=T12."水样测试") -> (queue out=w997:refnum<queue>, error out=w998:errorcluster)  [unwired: 3 in, 1 out]
                    n786 = Get Queue Status(queue=w997, error in (no error)=w998) -> (# elements in queue=w1001:i32)  [unwired: 1 in, 7 out]
                    n787 = Not Equal To 0?(x=w1001) -> (x != 0?=w1002:bool)
                    n788 = Greater Or Equal?(x=w999, y=1) -> (x >= y?=w1003:bool)
                    n789 = And(x=w1002, y=w1003) -> (x .and. y?=w995:bool)
                    n790 = case shown="真" w995 {
                      tunnel: [T6."读取数据" ("元素") T6."表格比对" ("元素")] -> w1005
                      frame False {
                      }
                      frame True {
                      }
                    }
                    n791 = Enqueue Element(queue=w1004, element=w1005) -> ()  [unwired: 2 in, 3 out]
                  }
                }
              }
            }
            n792 = case shown="假" w930 {
              tunnel: w931 -> [w976 _]
              tunnel: [w976 1 ("索引")] -> w935
              frame False {
              }
              frame True {
              }
            }
            "查询数据发送" <- TRUE
          }
          frame "数据处理" {
            n793 = local write "空闲时间"(0.0 ("空闲时间")) -> ()
            n794 = local read "心跳包"() -> (w1016:bool)
            n795 = Equal?(x=w1014, y="实时数据") -> (x = y?=w1012:bool)
            n796 = case shown="假" w1016 {
              tunnel: w1020 -> [w1023 _]
              tunnel: w1014 -> [w1022 _]
              frame False {
                n797 = call "插入单条数据.vi"("table输入"=w1022, "插入数据"=w1023) -> ()  [unwired: 8 in, 2 out]
              }
              frame True {
              }
            }
            n798 = Select(t=0, s=w1012, f=w1010) -> (s? t:f=w1011:i32)
            n799 = Enqueue Element(queue=w1019, element=T6."表格比对" ("元素"), timeout in ms (-1)=1000 ("超时毫秒(-1)")) -> ()  [unwired: 1 in, 3 out]
          }
        }
      }
      frame Error {
        n800 = Unbundle By Name(w1027) -> ("code"=w1026:i32)
        n801 = case shown="0, 默认" w1026 {
          tunnel: w1027 -> [w1032 w1042 w1071 w1095]
          tunnel: [w1038 w1055 w1084 w1095] -> w1031
          tunnel: w1025 -> [w1039 w1050 w1079 w1092]
          frame 0, Default {
            n802 = Flush Queue(queue=w1039) -> (queue out=w1037:refnum<queue>)  [unwired: 1 in, 2 out]
            n803 = global write "全局 数据发送重叠.vi" "掉线指示灯"(TRUE ("掉线指示灯")) -> ()
            n804 = local read "数据发送通道"() -> (w1034:enum16{"TCP", "VISA"})
            n805 = Enqueue Element(queue=w1037, element=T6."初始化" ("元素"), timeout in ms (-1)=1000 ("超时毫秒(-1)")) -> ()  [unwired: 1 in, 3 out]
            n806 = call "VISATCP组合选择发送.vi"("数据发送通道"=w1034, "命令"="close", "error in (no error)"=w1032) -> ("错误输出"=w1033:errorcluster)  [unwired: 9 in, 3 out]
            n807 = call <vilib>:"Clear Errors.vi"("error in (no error)"=w1033) -> ("error out"=w1038:errorcluster)  [unwired: 5 in, 1 out]
          }
          frame 63 {
            # "TCP服务器端口掉线"
            n808 = Flush Queue(queue=w1050) -> (queue out=w1051:refnum<queue>)  [unwired: 1 in, 2 out]
            n809 = global write "全局 数据发送重叠.vi" "掉线指示灯"(TRUE ("掉线指示灯")) -> ()
            n810 = property on="TCP服务端掉线计数" class="DigNum (严格)"() -> ("Value"=w1049:i32)  [unwired: 2 in, 2 out]
            n811 = property on="TCP服务端掉线计数" class="DigNum (严格)"() -> ("Value"=w1054:i32)  [unwired: 2 in, 2 out]
            n812 = local read "数据发送通道"() -> (w1044:enum16{"TCP", "VISA"})
            n813 = Increment(x=w1054) -> (x+1=w1052:i32)
            n814 = Less Or Equal?(x=w1049, y=1) -> (x <= y?=w1047:bool)
            n815 = Enqueue Element(queue=w1051, element=T6."初始化" ("元素"), timeout in ms (-1)=1000 ("超时毫秒(-1)")) -> ()  [unwired: 1 in, 3 out]
            n816 = case shown="真" w1047 {
              frame False {
                n817 = local write "TCP掉线时间节点"("TCP掉线时间节点") -> ()
                n818 = global write "全局 数据发送重叠.vi" "TCP掉线时间节点"("TCP掉线时间节点") -> ()
              }
              frame True {
                n819 = call <vilib>:"Application Directory.vi"() -> ("Application Directory"=w1066:path)
                n820 = Get Date/Time In Seconds() -> (seconds since 1Jan1904=w1068:timestamp)
                n821 = Build Path(base path=w1066, name or relative path="data\\Set.ini" ("名称或相对路径")) -> (appended path=w1067:path)
                n822 = Format Date/Time String(time format string (%c)="%Y%m%d%H%M%S%3u" ("时间格式字符串(%c)"), seconds (now)=w1068) -> (date/time string=w1070:string)  [unwired: 1 in]
                n823 = call "格式时间字符串.vi"("字符串"=w1070) -> ("连接的字符串"=w1058:string)  [unwired: 10 in]
                n824 = call <vilib>:"Open Config Data.vi"("configuration file path"=w1067) -> ("error out"=w1063:errorcluster, "refnum"=w1064:T8)  [unwired: 8 in, 1 out]
                n825 = local write "TCP掉线时间节点"(w1058) -> ()
                n826 = call-poly <vilib>:"Write Key.vi"("section"="掉线时间存储", "error in (no error)"=w1063, "value"=w1058, "key"="掉线时间", "refnum"=w1064) -> ("error out"=w1061:errorcluster, "refnum out"=w1062:T8)  [unwired: 4 in, 1 out]
                n827 = call <vilib>:"Close Config Data.vi"("error in (no error)"=w1061, "refnum"=w1062) -> ()  [unwired: 8 in, 2 out]
              }
            }
            n828 = property on="TCP服务端掉线计数" class="DigNum (严格)"("Value"=w1052) -> ()  [unwired: 2 in, 2 out]
            n829 = call "VISATCP组合选择发送.vi"("数据发送通道"=w1044, "命令"="close", "error in (no error)"=w1042) -> ("错误输出"=w1043:errorcluster)  [unwired: 9 in, 3 out]
            n830 = call <vilib>:"Clear Errors.vi"("error in (no error)"=w1043) -> ("error out"=w1055:errorcluster)  [unwired: 5 in, 1 out]
          }
          frame 54 {
            # "TCP服务器端口掉线"
            n831 = Flush Queue(queue=w1079) -> (queue out=w1080:refnum<queue>)  [unwired: 1 in, 2 out]
            n832 = global write "全局 数据发送重叠.vi" "掉线指示灯"(TRUE ("掉线指示灯")) -> ()
            n833 = property on="TCP服务端掉线计数" class="DigNum (严格)"() -> ("Value"=w1078:i32)  [unwired: 2 in, 2 out]
            n834 = property on="TCP服务端掉线计数" class="DigNum (严格)"() -> ("Value"=w1083:i32)  [unwired: 2 in, 2 out]
            n835 = local read "数据发送通道"() -> (w1073:enum16{"TCP", "VISA"})
            n836 = Increment(x=w1083) -> (x+1=w1081:i32)
            n837 = Less Or Equal?(x=w1078, y=1) -> (x <= y?=w1076:bool)
            n838 = Enqueue Element(queue=w1080, element=T6."初始化" ("元素"), timeout in ms (-1)=1000 ("超时毫秒(-1)")) -> ()  [unwired: 1 in, 3 out]
            n839 = case shown="真" w1076 {
              frame False {
                n840 = local read "TCP掉线时间节点"() -> (w1086:string)
                n841 = local write "TCP掉线时间节点"(w1086) -> ()
                n842 = global write "全局 数据发送重叠.vi" "TCP掉线时间节点"(w1086) -> ()
              }
              frame True {
                n843 = Get Date/Time In Seconds() -> (seconds since 1Jan1904=w1088:timestamp)
                n844 = Format Date/Time String(time format string (%c)="%Y%m%d%H%M%S%3u" ("时间格式字符串(%c)"), seconds (now)=w1088) -> (date/time string=w1090:string)  [unwired: 1 in]
                n845 = call "格式时间字符串.vi"("字符串"=w1090) -> ("连接的字符串"=w1087:string)  [unwired: 10 in]
                n846 = local write "TCP掉线时间节点"(w1087) -> ()
              }
            }
            n847 = property on="TCP服务端掉线计数" class="DigNum (严格)"("Value"=w1081) -> ()  [unwired: 2 in, 2 out]
            n848 = call "VISATCP组合选择发送.vi"("数据发送通道"=w1073, "命令"="close", "error in (no error)"=w1071) -> ("错误输出"=w1072:errorcluster)  [unwired: 9 in, 3 out]
            n849 = call <vilib>:"Clear Errors.vi"("error in (no error)"=w1072) -> ("error out"=w1084:errorcluster)  [unwired: 5 in, 1 out]
          }
          frame 56 {
            n850 = Flush Queue(queue=w1092) -> (queue out=w1093:refnum<queue>)  [unwired: 1 in, 2 out]
            n851 = Enqueue Element(queue=w1093, element=T6."读取数据" ("元素"), timeout in ms (-1)=1000 ("超时毫秒(-1)")) -> ()  [unwired: 1 in, 3 out]
          }
        }
        n852 = call <vilib>:"Clear Errors.vi"("error in (no error)"=w1031) -> ("error out"=w1030:errorcluster)  [unwired: 5 in, 1 out]
      }
    }
    n853 = Wait (ms)(milliseconds to wait=u32 300 ("等待时间（毫秒）")) -> ()  [unwired: 1 out]
  }
  n854 = flat-sequence {
    frame #0 {
      w1111 = "线程一自主部署站点保存"
      (unwired) path "C:/LabVIEW Project/builds/平台数据发送系统" ("Application Directory")
      w1173 = "" ("参数")
      w1098 = FALSE ("数据发送中断")
      w1144 = 0 ("数值")
      # "版本改动:增加了远程反控命令，和仪器端双向通讯，modbus TCP读写"
      # "ST参数选择"
      n855 = property class="VI"() -> ("Panel"=w1177:refnum<vi>)  [unwired: 2 in, 2 out]
      n856 = global write "全局 实时数据参数.vi" "参数"(w1173) -> ()
      n857 = local write "核查数据上传"(w1098) -> ()
      n858 = local write "查询数据发送"(w1098) -> ()
      n859 = local write "心跳包"(w1098) -> ()
      n860 = global write "全局 小时数据发送次数.vi" "小时数据发送次数"(w1144) -> ()
      n861 = local write "实时小时数据上传"(w1098) -> ()
      n862 = local write "系统状态改变"(w1098) -> ()
      n863 = property class="Pnl"(reference=w1177) -> ("Panes[]"=w1176:refnum<vi>[])  [unwired: 1 in, 2 out]
      n864 = global write "全局 实时数据参数.vi" "data"(string[][] [] ("data")) -> ()
      n865 = property on="窗格" class="Pane"("Origin"=T11 {"Horizontal"=0, "Vertical"=0} ("原点")) -> ()  [unwired: 2 in, 2 out]
      n866 = local write "空闲时间"(0.0 ("try")) -> ()
      n867 = global write "全局1.vi" "枚举"(enum16{"返回请求应答", "上传数据", "返回执行结果"}."返回请求应答" ("枚举")) -> ()
      n868 = global write "全局 实时数据参数.vi" "连接的字符串"(w1173) -> ()
      n869 = call <vilib>:"Application Directory.vi"() -> ("Application Directory"=w1171:path)
      n870 = for {
        tunnel: w1176 -> [w1188] mode=indexing
        tunnel: u32 15592941 ("窗格颜色") -> [w1189]
        n871 = property class="Pane"(reference=w1188, "PaneColor"=w1189) -> ()  [unwired: 1 in, 2 out]
      }
      n872 = Build Path(base path=w1171, name or relative path="data\\Set.ini" ("名称或相对路径")) -> (appended path=w1169:path)
      n873 = call <vilib>:"Open Config Data.vi"("configuration file path"=w1169) -> ("error out"=w1167:errorcluster, "refnum"=w1168:T8)  [unwired: 8 in, 1 out]
      n874 = call <vilib>:"Application Directory.vi"() -> ("Application Directory"=w1134:path)
      n875 = call-poly <vilib>:"Read Key.vi"("section"=w1111, "error in (no error)"=w1167, "key"="站点名称", "refnum"=w1168) -> ("error out"=w1164:errorcluster, "value"=w1125:string, "refnum out"=w1165:T8)  [unwired: 4 in, 1 out]
      n876 = call <vilib>:"Application Directory.vi"() -> ("Application Directory"=w1102:path)
      n877 = call <vilib>:"Application Directory.vi"() -> ("Application Directory"=w1130:path)
      n878 = call <vilib>:"Recursive File List.vi"("pattern"="*.exe", "Folder Path"=w1134) -> ("All Files in Dir"=w1142:path[])  [unwired: 5 in, 4 out]
      n879 = Build Path(base path=w1102, name or relative path="data\\sys.ini" ("名称或相对路径")) -> (appended path=w1100:path)
      n880 = local write "站点名称"(w1125) -> ()
      n881 = Build Path(base path=w1130, name or relative path="data\\background.jpg" ("名称或相对路径")) -> (appended path=w1129:path)
      n882 = call <vilib>:"Open Config Data.vi"("configuration file path"=w1100) -> ("error out"=w1106:errorcluster, "refnum"=w1105:T8)  [unwired: 8 in, 1 out]
      n883 = Index Array(array=w1142) -> (element=w1141:path)  [unwired: 1 in]
      n884 = Get Date/Time In Seconds() -> (seconds since 1Jan1904=w1181:timestamp)
      n885 = call <vilib>:"Read JPEG File.vi"("path to JPEG file"=w1129) -> ("error out"=w1127:errorcluster, "image data"=w1128:T13)  [unwired: 8 in, 1 out]
      n886 = vi-ref "断电保存全局.vi"() -> (w1104:refnum<vi>)
      n887 = Format Date/Time String(time format string (%c)="%Y%m%d%H%M%S%3u" ("时间格式字符串(%c)"), seconds (now)=w1181) -> (date/time string=w1180:string)  [unwired: 1 in]
      n888 = call-poly <vilib>:"Read Key.vi"("section"=w1111, "error in (no error)"=w1164, "key"="站点设备", "refnum"=w1165) -> ("error out"=w1161:errorcluster, "value"=w1124:string, "refnum out"=w1162:T8)  [unwired: 4 in, 1 out]
      n889 = File/Directory Info(path=w1141) -> (last mod=w1140:timestamp)  [unwired: 1 in, 6 out]
      n890 = call <vilib>:"FileVersionInfo.vi"("Application Path in"=w1141) -> ("error out"=w1126:errorcluster, "File Version Info"=w1137:string)  [unwired: 7 in, 2 out]
      n891 = call <userlib>:"Read Panel from INI__ogtk.vi"("error in (no error)"=w1106, "VI ref"=w1104, "refnum"=w1105) -> ("error out"=w1099:errorcluster, "refnum out"=w1103:T8)  [unwired: 7 in]
      n892 = property on="窗格" class="Pane"("BackgroundImage"=w1128) -> ()  [unwired: 2 in, 2 out]
      n893 = Format Date/Time String(time format string (%c)="\n%Y%m%d%H%M" ("时间格式字符串(%c)"), seconds (now)=w1140) -> (date/time string=w1136:string)  [unwired: 1 in]
      n894 = local write "站点设备"(w1124) -> ()
      n895 = case shown="错误" w1099 {
        frame No Error {
        }
        frame Error {
          n896 = global write "断电保存全局.vi" "数据发送协议"(enum16{"2005-212协议", "2017-212协议"}."2017-212协议" ("数据发送协议")) -> ()
          n897 = global write "断电保存全局.vi" "判断数据反馈"(TRUE ("判断数据反馈")) -> ()
          n898 = global write "断电保存全局.vi" "数据发送通道"(enum16{"TCP", "VISA"}."TCP" ("数据发送通道")) -> ()
        }
      }
      n899 = Search and Replace String(input string=w1180, search string="." ("搜索字符串")) -> (result string=w1178:string)  [unwired: 6 in, 3 out]
      n900 = call <vilib>:"Close Config Data.vi"("error in (no error)"=w1099, "refnum"=w1103) -> ()  [unwired: 8 in, 2 out]
      n901 = call-poly <vilib>:"Read Key.vi"("section"=w1111, "error in (no error)"=w1161, "key"="IP", "refnum"=w1162) -> ("error out"=w1158:errorcluster, "value"=w1123:string, "refnum out"=w1159:T8)  [unwired: 4 in, 1 out]
      n902 = Concatenate Strings("V" ("字符串"), w1137, w1136) -> (→"软件版本":string)
      n903 = local write "QN"(w1178) -> ()
      n904 = call <vilib>:"Simple Error Handler.vi"("error in (no error)"=w1126) -> ()  [unwired: 4 in, 5 out]
      n905 = call <vilib>:"Simple Error Handler.vi"("error in (no error)"=w1127) -> ()  [unwired: 4 in, 5 out]
      n906 = local write "IP"(w1123) -> ()
      n907 = call-poly <vilib>:"Read Key.vi"("section"=w1111, "error in (no error)"=w1158, "key"="PORT", "refnum"=w1159) -> ("error out"=w1154:errorcluster, "value"=w1122:string, "refnum out"=w1155:T8)  [unwired: 4 in, 1 out]
      n908 = call <vilib>:"Application Directory.vi"() -> ("Application Directory"=w1133:path)
      n909 = local write "PORT"(w1122) -> ()
      n910 = call "查询启动项.vi"("启动文件路径"=w1133) -> ("包含启动项"=w1132:bool)  [unwired: 9 in, 1 out]
      n911 = call-poly <vilib>:"Read Key.vi"("section"=w1111, "error in (no error)"=w1154, "key"="MN", "refnum"=w1155) -> ("error out"=w1118:errorcluster, "value"=w1121:string, "refnum out"=w1119:T8)  [unwired: 4 in, 1 out]
      n912 = local write "MN"(w1121) -> ()
      n913 = local write "开机启动"(w1132) -> ()
      n914 = call-poly <vilib>:"Read Key.vi"("section"=w1111, "error in (no error)"=w1118, "key"="PW", "refnum"=w1119) -> ("error out"=w1116:errorcluster, "value"=w1120:string, "refnum out"=w1117:T8)  [unwired: 4 in, 1 out]
      n915 = local write "PW"(w1120) -> ()
      n916 = call-poly <vilib>:"Read Key.vi"("section"=w1111, "error in (no error)"=w1116, "key"="VISA", "refnum"=w1117) -> ("error out"=w1112:errorcluster, "value"=w1114:string, "refnum out"=w1113:T8)  [unwired: 4 in, 1 out]
      n917 = local write "VISA resource name"(w1114) -> ()
      n918 = call-poly <vilib>:"Read Key.vi"("section"=w1111, "error in (no error)"=w1112, "key"="BAUDRATE", "refnum"=w1113) -> ("error out"=w1107:errorcluster, "value"=w1109:i32, "refnum out"=w1108:T8)  [unwired: 4 in, 1 out]
      n919 = local write "baud rate"(w1109) -> ()
      n920 = call-poly <vilib>:"Read Key.vi"("section"="系统编码选择", "error in (no error)"=w1107, "key"="系统编码", "refnum"=w1108) -> ("error out"=w1148:errorcluster, "value"=w1150:string, "refnum out"=w1149:T8)  [unwired: 4 in, 1 out]
      n921 = local write "系统编码选择框"(w1150) -> ()
      n922 = call-poly <vilib>:"Read Key.vi"("section"="掉线时间存储", "error in (no error)"=w1148, "key"="掉线时间", "refnum"=w1149) -> ("error out"=w1096:errorcluster, "value"=w1145:string, "refnum out"=w1097:T8)  [unwired: 4 in, 1 out]
      n923 = global write "全局 数据发送重叠.vi" "TCP掉线时间节点"(w1145) -> ()
      n924 = local write "TCP掉线时间节点"(w1145) -> ()
      n925 = call <vilib>:"Close Config Data.vi"("error in (no error)"=w1096, "refnum"=w1097) -> ()  [unwired: 8 in, 2 out]
      "TCP服务端掉线计数" <- w1144
    }
  }
  n926 = property class="VI"(reference=w38) -> ("Name"=w39:string)  [unwired: 1 in, 2 out]
  n927 = Open VI Reference(type specifier VI Refnum (for type only)=refnum<vi> refnum, vi path=w39, options=128 ("选项")) -> (vi reference=w41:refnum<vi>, error out=w43:errorcluster)  [unwired: 3 in]
  n928 = call-by-ref "?"(reference=w41, error in=w43) -> (reference out=w45:refnum<vi>, error out=w44:errorcluster)  [unwired: 11 in, 1 out]
  n929 = Close Reference(reference=w45, error in (no error)=w44) -> ()  [unwired: 1 out]
